vi "WS1050 36 DUT Reliability HD_Cycling Ver1.4.vi"() -> ()   [LabVIEW 2012]
uses:
  WS_VCAP Driver 029/Source/WSVCAP Shell/Type Defs/WSVCAP SHL I2C DUT Mask Mode Enum.ctl
  <vilib>/Utility/file.llb/Read From Spreadsheet File (DBL).vi
panel:
  out "VISA resource name out":refnum<visa-resource-name>="GPIB0::3::INSTR"
  out "error out 2":errorcluster={"status"=TRUE, "code"=-63192, "source"="niLvFpga_Open_PXI-7813R.vi"}
  in  "Reg1_Bit Cntrl":string[](array[string])=["01", "02", "04", "08", "10", "20", "40", "80", "03", "06", "0C", "D8", "33", "66", "CC", "07", "0E", "1C", "38", "70", "E0", "0F", "1E", "3C", "78", "F0", "1F", "3E", "7C", "F8", "3F", "7E", "FC", "7F", "FE", "FD", "FB", "F7", "EF", "DF", "BF", "7F", "FC", "F9", "F3", "E7", "CF", "9F", "3F", "F8", "F1", "E3", "C7", "8F", "1F", "F0", "E1", "C3", "87", "0F", "E0", "C1", "83", "07", "C0", "81", "03", "AA", "55", "00"]
  out "date string":string="5/19/2014"
  out "PS1 Out":refnum<visa-resource-name>
  out "Ke2000 Out":refnum<visa-resource-name>="GPIB0::9::INSTR"
  in  "VPI_Cmd":string[](array[string])=["00", "3B", "00"]
  in  "VPI Name":string[](array[string])=["All_Drivers OFF", "All Drivers ON", "All Drivers OFF2"]
  in  "Tab Control":T1(tab)
  in  "CP with DVA ON":i32(ring) items=["CP HDC 35V", "CP HDC 40.25V", "CP HDC 27.5V", "CP HDC 30.5V", "CP HDC 44V", "CP HDC 50V", "CP HDC 55V", "CP HDC 42.5V", "CP HDC 32V"]
  in  "No of Cmd":i64=2
  in  "Board#":string="BRD5"
  in  "Serial Number":string[][](table)=[["DUT", "SN"], ["DUT1", "1"], ["DUT2", "2"], ["DUT3", "3"], ["DUT4", "4"], ["DUT5", "5"], ["DUT6", "6"], ["DUT7", "7"], ["DUT8", "8"], ["DUT9", "9"], ["DUT10", "10"], ["DUT11", "11"], ["DUT12", "12"], ["DUT13", "13"], ["DUT14", "14"], ["DUT15", "15"], ["DUT16", "16"], ["DUT17", "17"], ["DUT18", "18"], ["DUT19", "19"], ["DUT20", "20"], ["DUT21", "21"], ["DUT22", "22"], ["DUT23", "23"], ["DUT24", "24"], ["DUT25", "25"], ["DUT26", "26"], ["DUT27", "27"], ["DUT28", "28"], ["DUT29", "29"], ["DUT30", "30"], ["DUT31", "31"], ["DUT32", "32"], ["DUT33", "33"], ["DUT34", "34"], ["DUT35", "35"], ["DUT36", "36"]]
  in  "SPI Clock Rate (Hz)":dbl=5000000.0 caption="Cycle Speed" format="%.1p Hz"
  in  "Wafer#":string="T7-EB"
  in  "File Name":string="CYC_WS1050_T7_EB_65C_40V_25DC_EMPTY_BRD5_151017_1"
  in  "TMN DC\\CAP Data Log File Path":path=path "C:/WS1050 36 DUT Data"
  in  "Test Program":string="WS1050 36 DUT Reliability HD_Cycling Ver1.4"
  out "Current Date":string="8/28/2014"
  out "Current Time":string="0950"
  in  "Start Date":string="10/21/2014"
  in  "Start Time":string="1542"
  in  "Comment":string="CYC65C40V"
  in  "OK Button":bool
  in  "Calibration":bool
  in  "Verify CP":bool
  in  "CP Setting":i32(ring) items=["CP OFF", "CP ON", "CP 35V", "CP 40V", "DVA ON", "DVA OFF", "REG1 ON", "REG1 OFF", "REG2 ON", "REG2 OFF", "REG3 ON", "REG3 OFF"]
  in  "Stop Calibration":bool
  in  "Set VDD":dbl=3.7 format="%.3g"
  in  "Command":string[](array[string])=["0702013B3B3B", "070201000000", "0702013B0000"]
  in  "Clock Rate (Hz)":dbl=1000000.0 caption="Meas Speed" format="%.1p Hz"
  out "AR  Measurent(Hz)":dbl
  in  "PS1 Source":refnum<visa-resource-name>="GPIB0::5::INSTR"
  in  "Ke2000":refnum<visa-resource-name>="GPIB0::9::INSTR"
  in  "CP to HD/Cycle":i32(ring)=1 items=["CP HDC 35V", "CP HDC 40.25V", "CP HDC 27.5V", "CP HDC 30.5V", "CP HDC 44V", "CP HDC 50V", "CP HDC 55V", "CP HDC 42.5V", "CP HDC 32V"]
  out "Simulate FPGA":bool
  out "Online":bool
  out "AR Cycling(Hz)":dbl=5000000.0
  in  "Ke2400":refnum<visa-resource-name>="GPIB0::3::INSTR"
  in  "Initialize AD7747":bool
  in  "DUT Mask Mode":T2=enum."All"
  in  "RFFE Slave Address":u8=7 caption="Slave Address" format="0x%02x"
  out "Activity Log":string="05/19/2014 -- 12:24:35.853::WSVCAP::APP::Application Started\n05/19/2014 -- 12:24:37.606::WSVCAP::WSVCAP SHL::WR I2C-REG:0x0A;MASK:0xFFFFFFFFFFFF;C1 DATA:22:22:22:22:22:22:22:22:22:22:22:22:22:22:22:22;C2 DATA:22:22:22:22:22:22:22:22:22:22:22:22:22:22:22:22;C3 DATA:22:22:22:22:22:22:22:22:22:22:22:22:22:22:22:22\r\n05/19/2014 -- 12:24:37.773::WSVCAP::WSVCAP SHL::WR I2C-ST:0,0,4,1\r\n05/19/2014 -- 12:24:37.903::WSVCAP::WSVCAP SHL::RD I2C-BYTES:4;ADD:0x00;MASK:0xFFFFFFFFFFFF\r\n05/19/2014 -- 12:24:38.045::WSVCAP::WSVCAP SHL::RD I2C:C1 DATA:2:2:2:2:2:2:2:2:2:2:2:2:2:2:2:2|A7:A9:AA:82:82:7F:82:81:82:81:83:82:81:82:82:81|46:36:BB:88:44:A3:E9:2B:32:20:ED:25:BB:3D:68:B|2C:6A:EB:A7:22:56:FE:CC:36:82:D7:B0:3B:48:F9:CC;C2 DATA:2:2:2:2:2:2:2:2:2:2:2:2:2:2:2:2|94:94:94:80:80:80:80:80:81:7E:7E:81:80:7E:80:80|47:33:15:82:62:B:E8:1C:D7:C3:7D:41:7C:B7:4C:2A|C4:B4:AE:8:1E:D1:4E:37:11:C0:6F:63:42:9D:63:B5;C3 DATA:2:2:2:2:2:2:2:2:2:2:2:2:2:2:2:2|95:95:95:81:81:7E:81:80:84:7D:80:83:81:7E:7F:80|AB:C4:14:B5:7B:52:DF:C9:79:5D:5F:30:99:31:1E:F4|6E:5C:F7:A8:C3:EB:7B:EF:33:92:89:77:4D:67:75:DD;STATUS:0:0:4:0\r\n05/19/2014 -- 12:24:38.046::WSVCAP::WSVCAP SHL::WR I2C-REG:0x0A;MASK:0xFFFFFFFFFFFF;C1 DATA:22:22:22:22:22:22:22:22:22:22:22:22:22:22:22:22;C2 DATA:22:22:22:22:22:22:22:22:22:22:22:22:22:22:22:22;C3 DATA:22:22:22:22:22:22:22:22:22:22:22:22:22:22:22:22\r\n05/19/2014 -- 12:24:38.089::WSVCAP::WSVCAP SHL::WR I2C-ST:0,0,4,1\r\n05/19/2014 -- 12:24:38.219::WSVCAP::WSVCAP SHL::RD I2C-BYTES:4;ADD:0x00;MASK:0xFFFFFFFFFFFF\r\n05/19/2014 -- 12:24:38.362::WSVCAP::WSVCAP SHL::RD I2C:C1 DATA:2:2:2:2:2:2:2:2:2:2:2:2:2:2:2:2|A7:AB:AA:82:82:82:83:83:82:82:82:82:7F:82:82:81|4B:32:96:83:3E:61:43:17:25:62:AB:4D:A2:40:2E:5|3C:76:2B:B4:EE:E4:A9:1A:AA:A:26:C7:21:2E:87:5B;C2 DATA:2:2:2:2:2:2:2:2:2:2:2:2:2:2:2:2|94:94:94:80:80:80:80:80:80:7F:80:81:80:80:7F:80|4A:32:19:7D:19:6C:79:46:61:7F:4B:B8:A5:30:F3:14|B4:70:A:8C:9C:DC:43:FA:1E:A:C6:21:A:A9:13:F3;C3 DATA:2:2:2:2:2:2:2:2:2:2:2:2:2:2:2:2|95:97:94:81:80:81:82:81:80:7E:81:84:7F:81:80:80|B2:32:D0:A7:9E:4C:AB:D4:EE:D9:F0:82:B7:91:7:FF|C1:91:B6:3D:D8:E:1B:4F:9F:6A:F1:6C:E7:3F:7:BA;STATUS:0:0:4:0\r\n05/19/2014 -- 12:24:38.364::WSVCAP::WSVCAP SHL::WR I2C-REG:0x0A;MASK:0xFFFFFFFFFFFF;C1 DATA:22:22:22:22:22:22:22:22:22:22:22:22:22:22:22:22;C2 DATA:22:22:22:22:22:22:22:22:22:22:22:22:22:22:22:22;C3 DATA:22:22:22:22:22:22:22:22:22:22:22:22:22:22:22:22\r\n05/19/2014 -- 12:24:38.406::WSVCAP::WSVCAP SHL::WR I2C-ST:0,0,4,1\r\n05/19/2014 -- 12:24:38.536::WSVCAP::WSVCAP SHL::RD I2C-BYTES:4;ADD:0x00;MASK:0xFFFFFFFFFFFF\r\n05/19/2014 -- 12:24:38.678::WSVCAP::WSVCAP SHL::RD I2C:C1 DATA:2:2:2:2:2:2:2:2:2:2:2:2:2:2:2:2|A7:A9:AB:82:82:81:82:82:82:82:82:82:82:82:82:81|46:71:4C:87:43:3D:7F:FC:25:4F:8E:54:97:3E:60:8C|AA:F4:1F:B5:CE:43:1F:36:9:87:9C:78:86:5:B6:8E;C2 DATA:2:2:2:2:2:2:2:2:2:2:2:2:2:2:2:2|94:94:94:80:7F:7F:80:80:80:80:80:81:80:80:80:80|49:36:18:7D:6E:C5:E4:3C:81:2E:41:D3:75:71:E3:72|E8:D3:E6:D1:E0:48:AE:D4:54:D:E8:8E:B4:41:68:4;C3 DATA:2:2:2:2:2:2:2:2:2:2:2:2:2:2:2:2|95:95:95:81:7F:7F:81:81:81:81:81:84:81:81:82:81|B3:F5:90:AB:82:69:7B:93:D0:77:E8:D5:E8:8C:84:E8|B9:AC:EE:2B:B6:71:8F:4A:74:31:56:BB:8A:B7:A0:C8;STATUS:0:0:4:0\r\n05/19/2014 -- 12:24:38.681::WSVCAP::WSVCAP SHL::WR I2C-REG:0x0A;MASK:0xFFFFFFFFFFFF;C1 DATA:22:22:22:22:22:22:22:22:22:22:22:22:22:22:22:22;C2 DATA:22:22:22:22:22:22:22:22:22:22:22:22:22:22:22:22;C3 DATA:22:22:22:22:22:22:22:22:22:22:22:22:22:22:22:22\r\n05/19/2014 -- 12:24:38.723::WSVCAP::WSVCAP SHL::WR I2C-ST:0,0,4,1\r\n05/19/2014 -- 12:24:38.854::WSVCAP::WSVCAP SHL::RD I2C-BYTES:4;ADD:0x00;MASK:0xFFFFFFFFFFFF\r\n05/19/2014 -- 12:24:38.996::WSVCAP::WSVCAP SHL::RD I2C:C1 DATA:2:2:2:2:2:2:2:2:2:2:2:2:2:2:2:2|A7:A9:AA:82:82:7F:83:81:82:81:84:82:7F:82:7F:82|43:FB:E:7F:3C:AD:35:35:26:A2:6C:21:4B:3D:8:6|63:9A:E1:F3:95:32:91:42:90:3C:78:1F:5C:D7:5F:D8;C2 DATA:2:2:2:2:2:2:2:2:2:2:2:2:2:2:2:2|94:94:94:80:80:80:80:80:81:80:7E:81:80:7E:7F:80|48:36:18:7F:5E:3D:69:83:DE:AE:A1:9E:31:AE:BB:96|15:A0:44:17:13:FD:CC:C8:6D:B2:EF:A7:C:C7:3B:F;C3 DATA:2:2:2:2:2:2:2:2:2:2:2:2:2:2:2:2|95:96:94:81:81:7E:82:80:84:80:80:84:7F:7E:7D:82|AD:3B:6D:A9:7C:57:9D:F5:7A:96:23:5C:36:2D:ED:5A|CD:46:DB:3B:C7:BD:70:60:33:B8:B:F7:63:A:51:4D;STATUS:0:0:4:0\r\n05/19/2014 -- 12:24:38.998::WSVCAP::WSVCAP SHL::WR I2C-REG:0x0A;MASK:0xFFFFFFFFFFFF;C1 DATA:22:22:22:22:22:22:22:22:22:22:22:22:22:22:22:22;C2 DATA:22:22:22:22:22:22:22:22:22:22:22:22:22:22:22:22;C3 DATA:22:22:22:22:22:22:22:22:22:22:22:22:22:22:22:22\r\n05/19/2014 -- 12:24:39.040::WSVCAP::WSVCAP SHL::WR I2C-ST:0,0,4,1\r\n05/19/2014 -- 12:24:39.170::WSVCAP::WSVCAP SHL::RD I2C-BYTES:4;ADD:0x00;MASK:0xFFFFFFFFFFFF\r\n05/19/2014 -- 12:24:39.311::WSVCAP::WSVCAP SHL::RD I2C:C1 DATA:2:2:2:2:2:2:2:2:2:2:2:2:2:2:2:2|A7:AA:AB:82:82:81:82:81:82:81:82:82:82:82:7F:82|44:F1:90:87:45:44:C8:2C:2C:F1:FC:1B:94:3B:3C:75|4A:49:95:19:99:73:64:3:23:24:F3:A2:5E:7F:C4:B6;C2 DATA:2:2:2:2:2:2:2:2:2:2:2:2:2:2:2:2|94:94:94:80:80:80:80:7F:80:80:7E:80:80:7E:7F:80|4C:36:17:7D:A8:9F:DE:C7:53:6D:8A:F4:41:A5:C6:E0|90:2E:24:C:D9:22:E4:76:3B:40:1D:53:33:B1:3E:4D;C3 DATA:2:2:2:2:2:2:2:2:2:2:2:2:2:2:2:2|95:97:95:81:81:7F:81:80:80:81:7F:82:81:7E:7D:82|AE:2B:A7:AB:CC:CD:A4:38:FD:17:80:F2:92:2D:45:C4|76:E5:D:B9:AD:B5:BA:8D:28:32:9E:42:B7:20:4A:D9;STATUS:0:0:4:0\r\n05/19/2014 -- 12:24:39.313::WSVCAP::WSVCAP SHL::WR I2C-REG:0x0A;MASK:0xFFFFFFFFFFFF;C1 DATA:22:22:22:22:22:22:22:22:22:22:22:22:22:22:22:22;C2 DATA:22:22:22:22:22:22:22:22:22:22:22:22:22:22:22:22;C3 DATA:22:22:22:22:22:22:22:22:22:22:22:22:22:22:22:22\r\n05/19/2014 -- 12:24:39.355::WSVCAP::WSVCAP SHL::WR I2C-ST:0,0,4,1\r\n05/19/2014 -- 12:24:39.486::WSVCAP::WSVCAP SHL::RD I2C-BYTES:4;ADD:0x00;MASK:0xFFFFFFFFFFFF\r\n05/19/2014 -- 12:24:39.628::WSVCAP::WSVCAP SHL::RD I2C:C1 DATA:2:2:2:2:2:2:2:2:2:2:2:2:2:2:2:2|A7:A9:AA:82:82:82:83:82:82:82:82:82:7F:82:7F:82|47:18:E4:87:3E:E7:6:65:25:92:37:38:A8:3E:89:85|7C:A7:7:2B:A3:7A:EC:EF:89:ED:F4:D3:D8:BC:3A:F5;C2 DATA:2:2:2:2:2:2:2:2:2:2:2:2:2:2:2:2|94:94:94:80:7F:80:80:7F:81:80:7E:80:80:80:81:80|49:37:17:80:76:25:6A:F8:DF:55:97:4D:B8:5B:2B:B1|13:E3:9A:3E:1A:2D:4F:B6:DB:E9:61:FA:8B:D6:9:CC;C3 DATA:2:2:2:2:2:2:2:2:2:2:2:2:2:2:2:2|95:95:95:81:7F:80:82:81:84:80:7F:81:80:81:7F:82|AF:93:3B:AF:5B:11:82:E4:7E:C3:2D:72:9:96:D9:A|DB:96:F2:10:5F:64:9A:C6:98:12:27:7D:10:D3:20:D9;STATUS:0:0:4:0\r\n05/19/2014 -- 12:24:40.132::WSVCAP::WSVCAP SHL::CLOSE\r\n"
  in  "C1 Cap DAC":u8=128 caption="B Data In" format="0x%02x"
  in  "C2 Cap DAC":u8=128 caption="B Data In" format="0x%02x"
  in  "C3 Cap DAC":u8=128 caption="B Data In" format="0x%02x"
  out "IDD Brd(uA)":string
  in  "Repeat Meas(s)":u32=900
  in  "Real No. From\nLookup Table":bool
  in  "Control Panel":T3={"Verify Socket"=FALSE, "HD/CYC"=FALSE, "E-CAL"=FALSE, "DVA"=FALSE, "VPI"=TRUE, "VSA"=TRUE, "HS"=TRUE}
  out "Verify Socket":bool
  out "HD/CYC":bool
  out "E-CAL":bool
  out "DVA":bool
  out "VPI":bool
  out "VSA":bool
  out "HS":bool
  in  "Lot#":string="WS1050"
  out "AD7747 Values":string[][](table)
  in  "Freq(Hz)":string="12K"
  in  "Reset P/S":bool
  in  "Test Sequences":i32(ring) items=["C1_C2_C3", "C2_C1_C3", "C3_C2_C1"]
  in  "WS1050/51":bool=TRUE
  in  "% Duty Cycle":string="25"
  in  "Cmd To HD":string="0702013B3B3B"
  in  "Post CMd Delay":dbl[](array[numeric])=[1.7e-05, 5.4e-05, 1.8e-05] min=0.0 max=0.5 format="%#.0p s"
  in  "Cmin/Act":bool=TRUE
  in  "CP to Meas":i32(ring)=1 items=["CP HDC 35V", "CP HDC 40.25V", "CP HDC 27.5V", "CP HDC 30.5V", "CP HDC 44V", "CP HDC 50V", "CP HDC 55V", "CP HDC 42.5V", "CP HDC 32V"]
  in  "CP VPI":i32(ring) items=["CP HDC 35V", "CP HDC 40.25V", "CP HDC 27.5V", "CP HDC 30.5V", "CP HDC 44V", "CP HDC 50V", "CP HDC 55V", "CP HDC 42.5V", "CP HDC 32V"]
  out "CAP_C1":string[][](table)
  out "NOM IDD OFF(uA)":string
  out "CAP_C2":string[][](table)
  out "CAP_C3":string[][](table)
  out "Total Time":u64
  in  "Set HD/Cycle \nto Complete":u64=5000000000
  out "No of HD/Cycle\nCompleted":u64
  out "Cycle Count":u64 min=1 max=4 step=1
  out "Loop \ncompleted":i32=1
  out "Previous Time":string="12:20:26 PM"
  out "STATUS":string="Idle...."
  out "Total Delta C2(pF)":string[](array[string])
  out "Total Delta C1(pF)":string[](array[string])
  out "Total Delta C3(pF)":string[](array[string])
  out "RB Reg for HD":string[](array[string])
  out "RB Reg for HD/Cycle":string[](array[string])
  out "VPI C2":string[][](table)
  out "VPI C3":string[][](table)
  out "NOM IDD ON (uA)":string
  out "IDD_HD/CYC (uA)":string="164.601255E+0"
  in  "stop During HD/Cycles":bool
  in  "stop":bool
  out "IDD Stdby(uA)":string="2.606990E+0"
  out "VPI C1":string[][](table)
  out "VSA_V1":string[][](table)
  out "VSA_V2":string[][](table)
  out "VSA_V3":string[][](table)
  in  "VSA Voltage(V)":dbl[](array[numeric])=[-10.0, 0.0, 10.0]
  in  "DC_Temp":i32=65
  in  "HD/CYC Temp":i32=65
  in  "Time All ON (s)":u32=120
  in  "Time All OFF (s)":u32=120
  in  "HD_DC (Min)":u64=259200
  out "LPs Count":i32
  in  "X Repeat":i32=100
  out "No LPs to RP":i32
  out "Run Loops":i32=1
  out "TTCompleted":u64=2000
  in  "TTF Completed":u64=5000000000
  out "% Delta C_T0":string[][](array[string])
  out "% Delta C":string[][](array[string])
  out "EFuse RB T0":string[](array[string])
  out "Current EFuse Read back":string[](array[string])
  out "EFuse Readback Status":bool[](array[boolean])
  in  "DeltaC Target Setting(pF)":dbl=7.375
  out "error out":errorcluster
  in  "error in (no error)":errorcluster
  in  "HD RP":dbl=60.0
  in  "Cycle RP":dbl=10000.0
  out "Min Plot_1":dbl[][](graph) caption="(Y) Multi Plot 2"
  out "Min Plot_2":dbl[][](graph) caption="(Y) Multi Plot 2"
  out "Min Plot_3":dbl[][](graph) caption="(Y) Multi Plot 2"
  in  "Debug":bool
  in  "No of Rows\nFrom Spread Sheet":i32
  in  "Plot Delta Cmin":bool=TRUE
  in  "Plot":T4(ring)
  in  "Bank C1":i32(ring) items=["C1", "C2", "C3", "D_C1", "D_C2", "D_C3"]
  in  "Bank C2":i32(ring)=1 items=["C1", "C2", "C3", "D_C1", "D_C2", "D_C3"]
  in  "Bank C3":i32(ring)=2 items=["C1", "C2", "C3", "D_C1", "D_C2", "D_C3"]
  # "Company:  WiSpry Inc\n20 Fairbanks Ste 198 Irvine CA 92618\n\nAuthor:  Andy V Tran\nCreated:  08/07/2015\nLabVIEW 2012 Pro\nTest Program:  WS1050 36 DUT Reliability HD_Cycling ver1.4\nFPGA: WS_VCAP Driver 029"
  # "Note for HD Duty Cycle:\n1.  Set time to start HD_DC (Min), default is 259200 (6 months) \n2.  Set Time for Duty Cycle ON/OFF, default setting is 2 minutes\n3.  No of Loops to RP = 3600s/(Time ALL ON(s) + Time ALL + OFF(s))\n4.  Set X Repeat = no of runs, default is 100 runs\n5.  Set TTF Completed to stop the test.\n\nVer 1.4 updated based on Ver1.3:\n1.  Updated P/S E3631A Driver\n2.  Updated KE2400 Driver\n3.  Updated CP to HD/Cycle"
  # "Minutes"
  # "X1000"
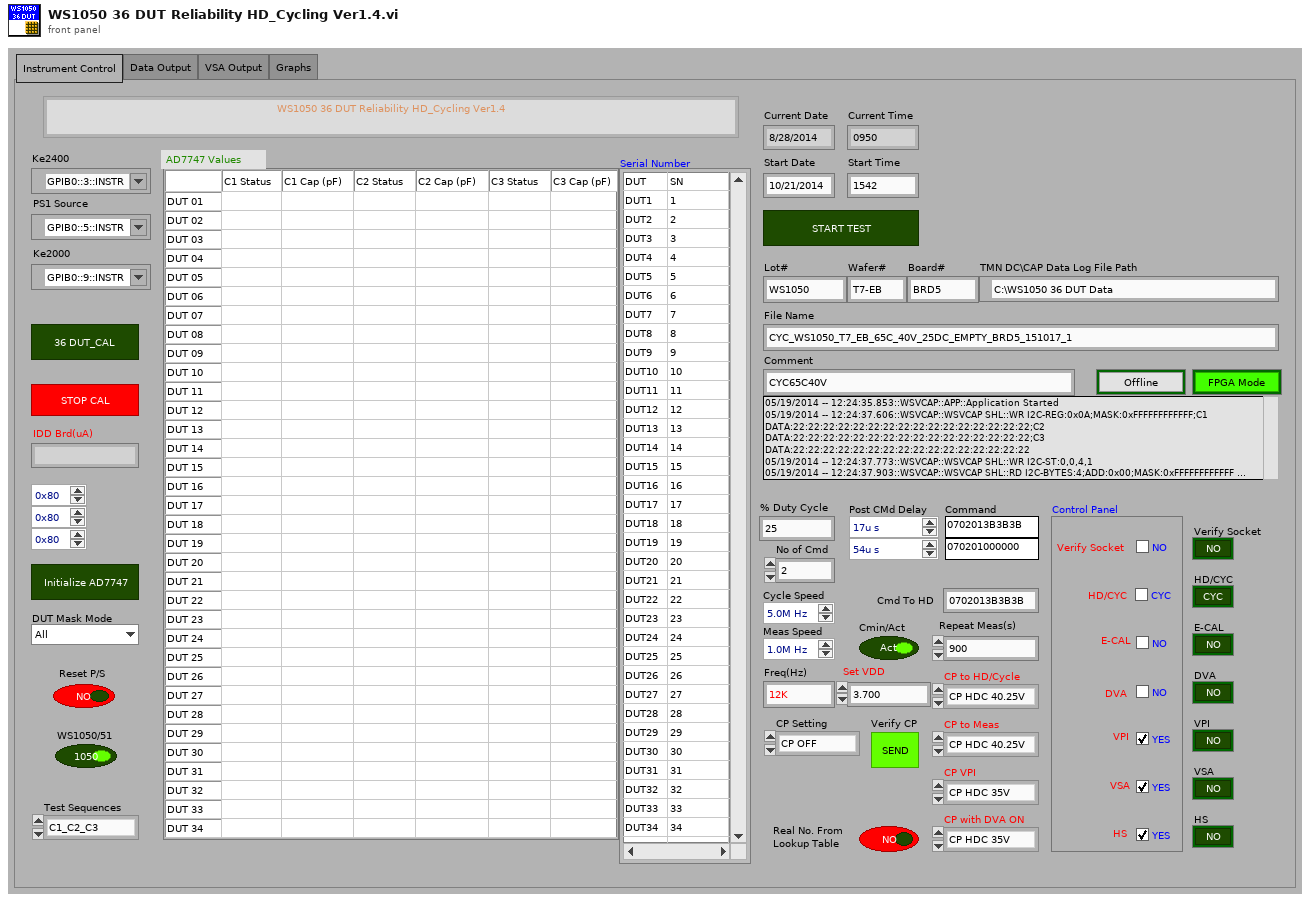
[diagram p1: front panel]
types:
  T1 = enum32{"Instrument Control", "Data Output", "VSA Output", "Graphs"}
  T2 = typedef "WSVCAP SHL I2C DUT Mask Mode Enum.ctl" = enum16{"Custom", "C1", "C2", "C3", "All"}
  T3 = cluster{"Verify Socket":bool, "HD/CYC":bool, "E-CAL":bool, "DVA":bool, "VPI":bool, "VSA":bool, "HS":bool}
  T4 = enum16{"ALL DUTs", "DUT 01", "DUT 02", "DUT 03", "DUT 04", "DUT 05", "DUT 06", "DUT 07", "DUT 08", "DUT 09", "DUT 10", "DUT 11", "DUT 12", "DUT 13", "DUT 14", "DUT 15", "DUT 16", "DUT 17", "DUT 18", "DUT 19", "DUT 20", "DUT 21", "DUT 22", "DUT 23", "DUT 24", "DUT 25", "DUT 26", "DUT 27", "DUT 28", "DUT 29", "DUT 30", "DUT 31", "DUT 32", "DUT 33", "DUT 34", "DUT 35", "DUT 36"}
  T5 = typedef "WSVCAP SHL Core System Cluster.ctl" = cluster{"Settings":T6, "FPGA Resource":tag, "Online":bool, "I2C Wait Ticks":u32, "SPI Wait Ticks":u32, "RFFE Wait Ticks":u32}
  T6 = typedef "WSVCAP SHL I2C Settings Cluster.ctl" = cluster{"FPGA Resource Name":string, "I2C Slave Address":u8, "I2C Clock Rate (Hz)":dbl, "SPI Clock Rate (Hz)":dbl, "RFFE Slave Address":u8, "RFFE Clock Rate (Hz)":dbl, "Simulate FPGA":bool, "C1 Cap DAC Default":u8, "C2 Cap DAC Default":u8, "C3 Cap DAC Default":u8}
  T7 = enum16{"Idle...", "Voltage 1", "Voltage 2", "Voltage 3"}[]
  T8 = cluster{"Test Program ":string, "Comment":string, "Data Out":string, "Data Out":string, "Data Out":string, string, "Data Out":string, "Data Out":string, "Data Out":string, "Freq(Hz)":string, "Board#":string}
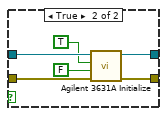
[diagram p2: hidden frame]
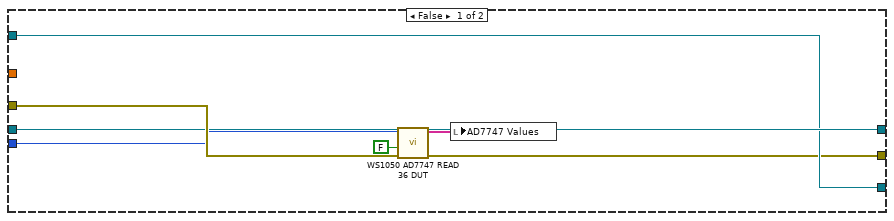
[diagram p10: hidden frame]
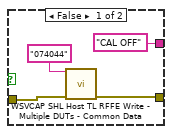
[diagram p11: hidden frame]
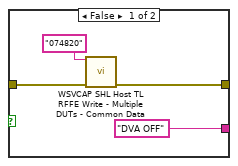
[diagram p12: hidden frame]
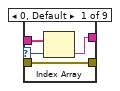
[diagram p13: hidden frame]
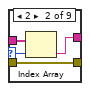
[diagram p14: hidden frame]
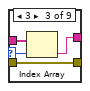
[diagram p15: hidden frame]
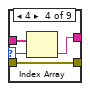
[diagram p16: hidden frame]
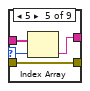
[diagram p17: hidden frame]
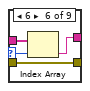
[diagram p18: hidden frame]
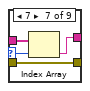
[diagram p19: hidden frame]
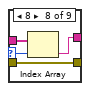
[diagram p20: hidden frame]
diagram:
  w25 = TRUE
  w29 = u16 0 items=["Off", "Moving Filter", "Repeating Filter"] ("Digital Filter (0: Off)")
  w30 = u16 7 items=["3.5 Digits"=4, "4.5 Digits"=5, "5.5 Digits"=6, "6.5 Digits"=7] ("Resolution (7: 6.5 digits)")
  n1 = case shown="True" w25 {
    tunnel: "error in (no error)" -> [w37 w38]
    tunnel: [w37 w45] -> w14
    frame False {
    }
    frame True {
      n2 = call "WSVCAP SHL Host TL Initialize.vi"("error in"=w38) -> ("error out"=w39:errorcluster)  [unwired: 13 in, 1 out]
      n3 = control-ref of="Activity Log"() -> (w41:refnum<vi>)
      n4 = call "ACT LG Activity Log Core.vi"("Display Ref"=w41, "Source"="WSVCAP", "Error In (no error)"=w39) -> ("Error Out"=w40:errorcluster)  [unwired: 11 in, 1 out]
      n5 = call "WSVCAP SHL Host TL Status Manager.vi"("error in"=w40) -> ("System Out"=w46:T5, "error out"=w45:errorcluster)  [unwired: 13 in]
      n6 = Unbundle By Name(w46) -> ("Online"=→"Online":bool, "Settings.Simulate FPGA"=→"Simulate FPGA":bool)
    }
  }
  n7 = case shown="True" TRUE {
    tunnel: w14 -> [w47 w52]
    tunnel: [w48 w51] -> w22
    tunnel: [w47 w50] -> w18
    tunnel: "Ke2400" -> [w48 w49]
    frame False {
    }
    frame True {
      n8 = VISA Write(VISA resource name=w49, write buffer="SOUR:FUNC VOLT;VOLT:MODE FIX;RANG 100;LEV 0.0;:SENS:FUNC \"CURR\";CURR:PROT 60E-3;RANG 100E-3;:OUTP ON", error in (no error)=w52) -> (VISA resource name out=w51:refnum<visa-resource-name>, error out=w50:errorcluster)  [unwired: 1 out]
    }
  }
  n9 = case shown="False" "Reset P/S" {
    tunnel: "PS1 Source" -> [w54 w61]
    tunnel: [w54 w59] -> w34
    tunnel: w14 -> [w55 w57]
    tunnel: [w55 w56] -> w13
    frame False {
    }
    frame True {
      n10 = call "Agilent 3631A Initialize.vi"("error in (no error)"=w57, "Default"=FALSE ("Reset? (T: Yes)"), "Reset"=TRUE ("ID Query? (T: Yes)"), "VISA resource name"=w61) -> ("error out"=w56:errorcluster, "VISA resource name out"=w59:refnum<visa-resource-name>)  [unwired: 6 in]
    }
  }
  n11 = call "Ke2000 Initialize.vi"("error in (no error)"=w14, "VISA resource name"="Ke2000") -> ("error out"=w31:errorcluster, "VISA resource name out"=w32:refnum<visa-resource-name>)  [unwired: 8 in]
  n12 = call "Ke2000 Configure DC Current.vi"("Resolution (7: 6.5 digits)"=w30, "Digital Filter (0: Off)"=w29, "Auto Range? (T: Auto)"=FALSE, "error in"=w31, "Custom Range (0 A)"=1.0, "VISA resource name"=w32) -> ("error out"=w15:errorcluster, "VISA resource name out"=w27:refnum<visa-resource-name>)  [unwired: 4 in]
  n13 = case shown="True" TRUE {
    tunnel: [_ w62] -> w36
    frame False {
    }
    frame True {
      n14 = call-poly <vilib>:"Read From Spreadsheet File.vi"("number of rows (all:-1)"=-1) -> ("all rows"=w62:dbl[][])  [unwired: 6 in, 4 out]
    }
  }
  n15 = Merge Errors(w18, w15, w13) -> (w23:errorcluster)
  n16 = while {
    tunnel: w23 -> [w70]
    tunnel: [w66] -> w4
    tunnel: w36 -> [w93]
    tunnel: w34 -> [w81]
    tunnel: w27 -> [w82]
    tunnel: [w91] -> w10
    tunnel: [w90] -> w5
    tunnel: w22 -> [w88]
    tunnel: [w87] -> w20
    tunnel: [FALSE ("stop")] -> w16
    i -> [w89]
    stop <- w94 stop-if-true
    n17 = case shown="0" w89 {
      tunnel: w70 -> [w104 w106]
      tunnel: [w103 w106] -> w84
      tunnel: "RFFE Slave Address" -> [w101 _]
      frame 0 {
        w97 = dbl[][] []
        w96 = "" ("uA")
        w98 = string[][] []
        w99 = string[] [] ("EFuse Read back")
        w105 = u64 0 ("No of HD/Cycle\nCompleted")
        n18 = local write "RB Reg for HD/Cycle"(w99) -> ()
        n19 = local write "Current EFuse Read back"(w99) -> ()
        n20 = local write "EFuse RB T0"(w99) -> ()
        n21 = local write "Total Delta C1(pF)"(w99) -> ()
        n22 = local write "Total Delta C2(pF)"(w99) -> ()
        n23 = local write "Total Delta C3(pF)"(w99) -> ()
        n24 = local write "No of HD/Cycle\nCompleted"(w105) -> ()
        n25 = local write "Cycle Count"(w105) -> ()
        n26 = local write "CAP_C2"(w98) -> ()
        n27 = local write "CAP_C1"(w98) -> ()
        n28 = local write "VPI C2"(w98) -> ()
        n29 = local write "VSA_V3"(w98) -> ()
        n30 = local write "VSA_V1"(w98) -> ()
        n31 = local write "NOM IDD OFF(uA)"(w96) -> ()
        n32 = local write "NOM IDD ON (uA)"(w96) -> ()
        n33 = local write "IDD Brd(uA)"(w96) -> ()
        n34 = local write "CAP_C3"(w98) -> ()
        n35 = local write "VSA_V2"(w98) -> ()
        n36 = local write "VPI C1"(w98) -> ()
        n37 = local write "VPI C3"(w98) -> ()
        n38 = local write "% Delta C"(w98) -> ()
        n39 = local write "% Delta C_T0"(w98) -> ()
        n40 = call "WSVCAP SHL Host TL RFFE Configure.vi"("RFFE Slave Address"=w101, "Clock Rate (Hz)"="Clock Rate (Hz)", "error in"=w104) -> ("Actual Rate (Hz)"=→"AR  Measurent(Hz)":dbl, "error out"=w103:errorcluster)  [unwired: 11 in]
        n41 = local write "Min Plot_3"(w97) -> ()
        n42 = local write "Min Plot_1"(w97) -> ()
        n43 = local write "Min Plot_2"(w97) -> ()
      }
      frame 1, Default {
      }
    }
    n44 = while {
      tunnel: ["stop"] -> w86
      tunnel: w84 -> [w134]
      tunnel: [w126] -> w78
      tunnel: w81 -> [w133]
      tunnel: w82 -> [w128]
      tunnel: [w129] -> w80
      tunnel: [w127] -> w79
      tunnel: [w124] -> w77
      tunnel: [w123] -> w76
      tunnel: [w122] -> w75
      tunnel: [w121] -> w74
      tunnel: [w120] -> w73
      tunnel: [w119] -> w72
      tunnel: [w118] -> w71
      tunnel: ["Command"] -> w69
      tunnel: ["Post CMd Delay"] -> w68
      tunnel: "Set VDD" -> [w108]
      stop <- w141 stop-if-true
      # "Set Date & Time to Start Test"
      n45 = case shown="True" "Initialize AD7747" {
        tunnel: w134 -> [w150 w156]
        tunnel: [w150 w152] -> w117
        tunnel: w133 -> [w149 w154]
        tunnel: [w149 w153] -> w132
        tunnel: w108 -> [_ w151]
        frame False {
        }
        frame True {
          w157 = T7 [enum."Voltage 2", enum."Voltage 3", enum."Voltage 1"] items=["Idle...", "Voltage 1", "Voltage 2", "Voltage 3"]
          n46 = for {
            tunnel: w154 -> [w167]
            tunnel: w157 -> [w165] mode=indexing
            tunnel: [w164] -> w153
            shift-right: [w161] -> w155
            shift-left: w156 -> [w168]
            tunnel: w151 -> [w158]
            n47 = call "E3631A_Voltage Controller updated.vi"("VISA resource name"=w167, "I_VDD(A)"=0.5, "Channel Controller"=w165, "Voltage 1"=w158, "Voltage 2"=3.3, "error in (no error)"=w168, "I_3.3V (A)"=0.5) -> ("VISA resource name out"=w164:refnum<visa-resource-name>, "error out"=w160:errorcluster)  [unwired: 7 in]
            n48 = call "Delay.vi"("milliseconds to wait"=u32 100, "error in (no error)"=w160) -> ("error out"=w161:errorcluster)  [unwired: 9 in]
          }
          n49 = call "WS1050_AD7747_Init 36DUT.vi"("error in"=w155) -> ("error out"=w152:errorcluster)  [unwired: 10 in]
        }
      }
      n50 = call "Time_stamp.vi"() -> ("date/time string"=w146:string, "date string"=w148:string)  [unwired: 2 in]
      "Current Date" <- w148
      "Current Time" <- w146
      n51 = Equal?(x=w148, y="Start Date") -> (x = y?=w144:bool)
      n52 = Equal?(x=w146, y="Start Time") -> (x = y?=w143:bool)
      n53 = And(x=w144, y=w143) -> (x .and. y?=w140:bool)
      n54 = Compound Arithmetic op=OR(w140, "OK Button", "stop") -> (w141:bool)
      n55 = case shown="True" "Calibration" {
        tunnel: w117 -> [w199 w217]
        tunnel: [w193 w214] -> w115
        tunnel: w132 -> [w198 w213]
        tunnel: "DUT Mask Mode" -> [w197 w209]
        tunnel: [w198 w208] -> w130
        tunnel: w128 -> [w196 w204]
        tunnel: [w196 w201] -> w127
        tunnel: w108 -> [_ w200]
        frame False {
          n56 = call "WS1050 AD7747 READ 36 DUT.vi"("error in"=w199, "Log (T)"=FALSE, "DUT Mask Mode (All)"=w197) -> ("error out"=w193:errorcluster, "AD7747 Values"=w194:string[][])  [unwired: 7 in]
          n57 = local write "AD7747 Values"(w194) -> ()
        }
        frame True {
          n58 = flat-sequence {
            tunnel: w217 -> [w227]
            tunnel: [w222] -> w216
            tunnel: w213 -> [w226]
            tunnel: [w225] -> w212
            tunnel: w209 -> [w224]
            tunnel: [w224] -> w210
            tunnel: w204 -> [w220]
            tunnel: [w219] -> w203
            tunnel: w200 -> [w218]
            tunnel: w216 -> [w251]
            tunnel: [w250] -> w215
            tunnel: w212 -> [w249]
            tunnel: [w249] -> w211
            tunnel: w210 -> [w248]
            tunnel: "C1 Cap DAC" -> [w244]
            tunnel: "C2 Cap DAC" -> [w243]
            tunnel: "C3 Cap DAC" -> [w242]
            tunnel: w203 -> [w241]
            tunnel: [w241] -> w202
            tunnel: w215 -> [w260]
            tunnel: [w263] -> w214
            tunnel: w211 -> [w262]
            tunnel: [w259] -> w208
            tunnel: w202 -> [w258]
            tunnel: [w258] -> w201
            frame #0 {
              w228 = T7 [enum."Voltage 2", enum."Voltage 3", enum."Voltage 1"] items=["Idle...", "Voltage 1", "Voltage 2", "Voltage 3"]
              n59 = for {
                tunnel: w226 -> [w239]
                tunnel: w228 -> [w237] mode=indexing
                tunnel: [w236] -> w225
                shift-right: [w234] -> w221
                shift-left: w227 -> [w240]
                tunnel: w218 -> [w230]
                n60 = call "E3631A_Voltage Controller updated.vi"("VISA resource name"=w239, "I_VDD(A)"=0.5, "Channel Controller"=w237, "Voltage 1"=w230, "Voltage 2"=3.3, "error in (no error)"=w240, "I_3.3V (A)"=0.5) -> ("VISA resource name out"=w236:refnum<visa-resource-name>, "error out"=w233:errorcluster)  [unwired: 7 in]
                n61 = call "Delay.vi"("milliseconds to wait"=u32 100, "error in (no error)"=w233) -> ("error out"=w234:errorcluster)  [unwired: 9 in]
              }
              n62 = call "Ke2000 Single Reading.vi"("error in (no error)"=w221, "VISA resource name"=w220) -> ("error out"=w222:errorcluster, "VISA resource name out"=w219:refnum<visa-resource-name>, "uA"=→"IDD Brd(uA)":string)  [unwired: 5 in, 2 out]
              n63 = One Button Dialog(message="Please verify all sockets should be empty...") -> ()  [unwired: 1 in, 1 out]
            }
            frame #1 {
              n64 = call "WS1050 CAPDAC Setting.vi"("DUT Mask Mode (All)"=w248, "error in"=w251, "C3 Cap DAC"=w242, "C2 Cap DAC"=w243, "C1 Cap DAC"=w244) -> ("error out"=w246:errorcluster)  [unwired: 5 in, 1 out]
              n65 = call "WS1050 OFFSET CAL.vi"("error in"=w246, "OFFSET CAL"=TRUE ("Read?")) -> ("error out"=w245:errorcluster)  [unwired: 8 in, 1 out]
              n66 = while {
                tunnel: w245 -> [w257]
                tunnel: [w256] -> w250
                tunnel: w248 -> [w254]
                stop <- "Stop Calibration" stop-if-true
                n67 = call "WS1050 AD7747 READ 36 DUT.vi"("error in"=w257, "Log (T)"=FALSE, "DUT Mask Mode (All)"=w254) -> ("error out"=w256:errorcluster, "AD7747 Values"=→"AD7747 Values":string[][])  [unwired: 7 in]
              }
            }
            frame #2 {
              w261 = T7 [enum."Voltage 2", enum."Voltage 3", enum."Voltage 1"] items=["Idle...", "Voltage 1", "Voltage 2", "Voltage 3"]
              n68 = for {
                tunnel: w262 -> [w275]
                tunnel: w261 -> [w272] mode=indexing
                tunnel: [w271] -> w259
                shift-right: [w267] -> w263
                shift-left: w260 -> [w273]
                n69 = call "E3631A_Voltage Controller updated.vi"("VISA resource name"=w275, "I_VDD(A)"=0.5, "Channel Controller"=w272, "Voltage 1"=0.0, "Voltage 2"=3.3, "error in (no error)"=w273, "I_3.3V (A)"=0.5) -> ("VISA resource name out"=w271:refnum<visa-resource-name>, "error out"=w266:errorcluster)  [unwired: 7 in]
                n70 = call "Delay.vi"("milliseconds to wait"=u32 100, "error in (no error)"=w266) -> ("error out"=w267:errorcluster)  [unwired: 9 in]
              }
              n71 = One Button Dialog(message="Calibration Completed....") -> ()  [unwired: 1 in, 1 out]
            }
          }
        }
      }
      n72 = local write "stop During HD/Cycles"(FALSE ("stop During HD/Cycles")) -> ()
      n73 = call "Control Panel.vi"("error in (no error)"=w117, "Control Panel"="Control Panel") -> ("error out"=w114:errorcluster, "VPI"=w120:bool, "DVA"=w121:bool, "E-CAL"=w122:bool, "VSA"=w119:bool, "HD/CYC"=w123:bool, "HS"=w118:bool, "Verify Socket"=w124:bool)  [unwired: 2 in]
      "Verify Socket" <- w124
      "E-CAL" <- w122
      "VPI" <- w120
      "VSA" <- w119
      "HS" <- w118
      "HD/CYC" <- w123
      "DVA" <- w121
      n74 = Merge Errors(w114, w115) -> (w116:errorcluster)
      n75 = case shown="True" "Verify CP" {
        tunnel: [w169 w174] -> w126
        tunnel: w130 -> [w170 w177]
        tunnel: [w170 w175] -> w129
        tunnel: w116 -> [w169 w173]
        tunnel: w108 -> [_ w171]
        frame False {
        }
        frame True {
          w178 = T7 [enum."Voltage 2", enum."Voltage 3", enum."Voltage 1"] items=["Idle...", "Voltage 1", "Voltage 2", "Voltage 3"]
          # "Verify CP"
          n76 = for {
            tunnel: w177 -> [w191]
            tunnel: w178 -> [w189] mode=indexing
            shift-right: [w187] -> w176
            shift-left: w173 -> [w192]
            tunnel: [w185] -> w175
            tunnel: w171 -> [w182]
            n77 = call "E3631A_Voltage Controller updated.vi"("VISA resource name"=w191, "I_VDD(A)"=0.5, "Channel Controller"=w189, "Voltage 1"=w182, "Voltage 2"=3.3, "error in (no error)"=w192, "I_3.3V (A)"=0.5) -> ("VISA resource name out"=w185:refnum<visa-resource-name>, "error out"=w188:errorcluster)  [unwired: 7 in]
            n78 = call "Delay.vi"("milliseconds to wait"=u32 100, "error in (no error)"=w188) -> ("error out"=w187:errorcluster)  [unwired: 9 in]
          }
          n79 = Index Array(array=string[] ["074000", "074040", "07476F", "074776", "074800", "074820", "07413B", "074100", "07423B", "074200", "07433B", "074300"], index="CP Setting") -> (element=w179:string)
          n80 = call "WSVCAP SHL Host TL RFFE Write - Multiple DUTs - Common Data.vi"("Data Out"=w179, "error in"=w176, "Log (T)"=FALSE) -> ("error out"=w174:errorcluster)  [unwired: 12 in]
        }
      }
      n81 = Array Subset(array="Post CMd Delay", length="No of Cmd") -> (w112:dbl[])  [unwired: 1 in]
      n82 = Array Subset(array="Command", length="No of Cmd") -> (w113:string[])  [unwired: 1 in]
      n83 = property on="Post CMd Delay" class="Arr (strict)"("Number of Rows"="No of Cmd") -> ()  [unwired: 2 in, 2 out]
      n84 = local write "Command"(w113) -> ()
      n85 = local write "Post CMd Delay"(w112) -> ()
      n86 = property on="Command" class="Arr (strict)"("Number of Rows"="No of Cmd") -> ()  [unwired: 2 in, 2 out]
      n87 = Wait Until Next ms Multiple(millisecond multiple=u32 100) -> ()  [unwired: 1 out]
    }
    n88 = case shown="False" w86 {
      tunnel: w78 -> [w336 w2007]
      tunnel: [w321 w2007] -> w66
      tunnel: w93 -> [w337 _]
      tunnel: w80 -> [w335 w2005]
      tunnel: w79 -> [w327 w2006]
      tunnel: [w333 w2006] -> w91
      tunnel: [w331 w2005] -> w90
      tunnel: w88 -> [w324 w2004]
      tunnel: [w320 w2004] -> w87
      tunnel: "RFFE Slave Address" -> [w315 _]
      tunnel: [FALSE ("stop During HD/Cycles") FALSE ("stop During HD/Cycles")] -> _
      tunnel: w77 -> [w291 _]
      tunnel: w76 -> [w290 _]
      tunnel: w75 -> [w289 _]
      tunnel: w74 -> [w288 _]
      tunnel: w73 -> [w287 _]
      tunnel: w72 -> [w286 _]
      tunnel: w71 -> [w285 _]
      tunnel: w69 -> [w279 _]
      tunnel: w68 -> [w278 _]
      tunnel: "Set VDD" -> [w277 _]
      tunnel: [w276 _] -> w64
      frame False {
        w316 = u64 0 ("Total Completed")
        w296 = u32 100 ("milliseconds to wait")
        w332 = T7 [enum."Voltage 2", enum."Voltage 3", enum."Voltage 1"] items=["Idle...", "Voltage 1", "Voltage 2", "Voltage 3"]
        w334 = T7 [enum."Voltage 2", enum."Voltage 3", enum."Voltage 1"] items=["Idle...", "Voltage 1", "Voltage 2", "Voltage 3"]
        # "VSA"
        # "HS"
        # "HD/CYC"
        # "DVA"
        # "E-CAL"
        # "VPI"
        # "Verify Socket"
        n89 = for {
          tunnel: w336 -> [w2002]
          tunnel: w335 -> [w2001]
          tunnel: w334 -> [w1999] mode=indexing
          tunnel: [w1995] -> w329
          tunnel: [w1998] -> w319
          tunnel: w277 -> [w1992]
          n90 = call "E3631A_Voltage Controller updated.vi"("VISA resource name"=w2001, "I_VDD(A)"=0.5, "Channel Controller"=w1999, "Voltage 1"=w1992, "Voltage 2"=3.3, "error in (no error)"=w2002, "I_3.3V (A)"=0.5) -> ("VISA resource name out"=w1998:refnum<visa-resource-name>, "error out"=w1996:errorcluster)  [unwired: 7 in]
          n91 = call "Delay.vi"("milliseconds to wait"=u32 100, "error in (no error)"=w1996) -> ("error out"=w1995:errorcluster)  [unwired: 9 in]
        }
        n92 = local write "TTCompleted"(w316) -> ()
        n93 = local write "Total Time"(w316) -> ()
        n94 = call "WSVCAP SHL Host TL RFFE Write - Multiple DUTs - Common Data.vi"("Data Out"="074000", "error in"=w329, "Log (T)"=FALSE) -> ("error out"=w330:errorcluster)  [unwired: 12 in]
        n95 = local read "IDD Brd(uA)"() -> (w304:string)
        n96 = call "Delay.vi"("milliseconds to wait"=w296, "error in (no error)"=w330) -> ("error out"=w328:errorcluster)  [unwired: 9 in]
        n97 = call "Ke2000 Single Reading.vi"("error in (no error)"=w328, "VISA resource name"=w327) -> ("error out"=w305:errorcluster, "VISA resource name out"=w326:refnum<visa-resource-name>, "uA"=w307:string)  [unwired: 5 in, 2 out]
        n98 = call "Substration.vi"("error in (no error)"=w305, "Input2"=w304, "Input1"=w307) -> ("error out"=w281:errorcluster, "In1 - In2"=w306:string)  [unwired: 7 in]
        "IDD Stdby(uA)" <- w306
        n99 = case shown="True" w290 {
          tunnel: [1 ("X Repeat") w409] -> w318
          frame False {
          }
          frame True {
            n100 = local read "X Repeat"() -> (w409:i32)
          }
        }
        n101 = call "WSVCAP SHL Host TL RFFE Write - Multiple DUTs - Common Data.vi"("Data Out"="074040", "error in"=w281, "Log (T)"=FALSE) -> ("error out"=w280:errorcluster)  [unwired: 12 in]
        n102 = call "Delay.vi"("milliseconds to wait"=w296, "error in (no error)"=w280) -> ("error out"=w313:errorcluster)  [unwired: 9 in]
        n103 = case shown="True" w288 {
          tunnel: w313 -> [w360 w369]
          tunnel: [w359 w367] -> w311
          tunnel: ["DVA OFF" ("Data Out") "DVA ON" ("Data Out")] -> w312
          frame False {
            n104 = call "WSVCAP SHL Host TL RFFE Write - Multiple DUTs - Common Data.vi"("Data Out"="074820", "error in"=w360) -> ("error out"=w359:errorcluster)  [unwired: 13 in]
          }
          frame True {
            n105 = call "WSVCAP SHL Host TL RFFE Write - Multiple DUTs - Common Data.vi"("Data Out"="074800", "error in"=w369, "Log (T)"=FALSE) -> ("error out"=w365:errorcluster)  [unwired: 12 in]
            n106 = case shown="1" "CP with DVA ON" {
              selector: "CP with DVA ON" -> [w375 w379 w383 w387 w391 w395 w399 w403 w407]
              tunnel: [w374 w378 w382 w386 w390 w394 w398 w402 w405] -> w362
              tunnel: [w373 w377 w381 w385 w389 w393 w397 w401 w406] -> w364
              tunnel: w365 -> [w373 w377 w381 w385 w389 w393 w397 w401 w406]
              tunnel: string[] ["07476F", "074776", "074765", "074769", "07477B", "07477C", "07477D", "074779", "07476B"] -> [w372 w376 w380 w384 w388 w392 w396 w400 w404]
              frame 0, Default {
                n107 = Index Array(array=w372, index=w375) -> (element=w374:string)
              }
              frame 2 {
                n108 = Index Array(array=w376, index=w379) -> (element=w378:string)
              }
              frame 3 {
                n109 = Index Array(array=w380, index=w383) -> (element=w382:string)
              }
              frame 4 {
                n110 = Index Array(array=w384, index=w387) -> (element=w386:string)
              }
              frame 5 {
                n111 = Index Array(array=w388, index=w391) -> (element=w390:string)
              }
              frame 6 {
                n112 = Index Array(array=w392, index=w395) -> (element=w394:string)
              }
              frame 7 {
                n113 = Index Array(array=w396, index=w399) -> (element=w398:string)
              }
              frame 8 {
                n114 = Index Array(array=w400, index=w403) -> (element=w402:string)
              }
              frame 1 {
                n115 = Index Array(array=w404, index=w407) -> (element=w405:string)
              }
            }
            n116 = call "WSVCAP SHL Host TL RFFE Write - Multiple DUTs - Common Data.vi"("Data Out"=w362, "error in"=w364, "Log (T)"=FALSE) -> ("error out"=w367:errorcluster)  [unwired: 12 in]
          }
        }
        n117 = for {
          N: 36 -> [_]
          tunnel: "Serial Number" -> [w342]
          tunnel: [w340] -> w293 mode=indexing
          i -> [w339]
          n118 = Increment(x=w339) -> (x+1=w338:i32)
          n119 = Index Array(array=w342, index (row)=w338, index (col)=1 ("disabled index (col)")) -> (element=w340:string)
        }
        n120 = Not(x=w285) -> (.not. x?=w292:bool)
        n121 = Number To Fractional String(number=w277, precision (6)=i16 2) -> (F-format string=w309:string)  [unwired: 2 in]
        n122 = call "Delay.vi"("milliseconds to wait"=w296, "error in (no error)"=w311) -> ("error out"=w299:errorcluster)  [unwired: 9 in]
        n123 = case shown="True" w289 {
          tunnel: w299 -> [w346 w348]
          tunnel: [w343 w347] -> w298
          tunnel: ["CAL OFF" ("Data Out") "CAL ON" ("Data Out")] -> w300
          frame False {
            n124 = call "WSVCAP SHL Host TL RFFE Write - Multiple DUTs - Common Data.vi"("Data Out"="074044", "error in"=w346) -> ("error out"=w343:errorcluster)  [unwired: 13 in]
          }
          frame True {
            n125 = for {
              tunnel: string[] ["074900", "074920", "074900"] -> [w356] mode=indexing
              tunnel: w348 -> [w353]
              tunnel: [w352] -> w347
              n126 = call "WSVCAP SHL Host TL RFFE Write - Multiple DUTs - Common Data.vi"("Data Out"=w356, "error in"=w353, "Log (T)"=FALSE) -> ("error out"=w355:errorcluster)  [unwired: 12 in]
              n127 = call "Delay.vi"("milliseconds to wait"=u32 10, "error in (no error)"=w355) -> ("error out"=w352:errorcluster)  [unwired: 9 in]
            }
          }
        }
        n128 = for {
          N: w318 -> [_]
          tunnel: w337 -> [w447]
          tunnel: [w443] -> w333
          tunnel: w306 -> [w442]
          tunnel: w326 -> [w441]
          tunnel: "TMN DC\\CAP Data Log File Path" -> [w440]
          tunnel: w324 -> [w438]
          tunnel: [w437] -> w322
          tunnel: w319 -> [w413]
          shift-right: [w432] -> _
          shift-left: u64 0 -> [w434]
          tunnel: w290 -> [w431]
          tunnel: w315 -> [w426]
          tunnel: w315 -> [w425]
          tunnel: w312 -> [w424]
          tunnel: w309 -> [w423]
          tunnel: [w422] -> w303
          tunnel: w300 -> [w421]
          tunnel: w298 -> [w420]
          tunnel: w288 -> [w419]
          tunnel: w291 -> [w418]
          tunnel: w287 -> [w417]
          tunnel: w292 -> [w416]
          tunnel: w286 -> [w415]
          tunnel: w293 -> [w414]
          tunnel: [w413] -> w282
          tunnel: w279 -> [w412]
          tunnel: w278 -> [w411]
          tunnel: [w410] -> w276
          i -> [w430]
          stop <- w410 stop-if-true
          n129 = while {
            tunnel: w447 -> [w668]
            tunnel: w440 -> [w679]
            tunnel: "Lot#" -> [w678]
            tunnel: "Wafer#" -> [w677]
            tunnel: w414 -> [w676]
            tunnel: "Test Program" -> [w675]
            tunnel: w414 -> [w674]
            tunnel: "Comment" -> [w673]
            tunnel: "Lot#" -> [w672]
            tunnel: "Wafer#" -> [w671]
            tunnel: w441 -> [w667]
            tunnel: [w670] -> w443
            tunnel: w442 -> [w666]
            tunnel: w438 -> [w663]
            tunnel: [w662] -> w437
            tunnel: [w570] -> w428
            tunnel: w430 -> [w608]
            tunnel: [w599] -> w432
            tunnel: w434 -> [w598]
            shift-right: [w597] -> _
            shift-left: u64 0 -> [w494]
            tunnel: [w596] -> w427
            tunnel: w431 -> [w594]
            tunnel: w426 -> [w569]
            tunnel: w425 -> [w567]
            tunnel: w424 -> [w517]
            tunnel: w423 -> [w515]
            tunnel: [w491] -> w422
            tunnel: w421 -> [w498]
            tunnel: w420 -> [w497]
            tunnel: w419 -> [w496]
            tunnel: w418 -> [w488]
            tunnel: w417 -> [w487]
            tunnel: w416 -> [w482]
            tunnel: w415 -> [w476]
            tunnel: w412 -> [w452]
            tunnel: w411 -> [w451]
            i -> [w595]
            stop <- w609 stop-if-true
            n130 = case shown="8" "CP to HD/Cycle" {
              selector: "CP to HD/Cycle" -> [w683 w688 w693 w698 w703 w708 w713 w718 w722]
              tunnel: string[] ["07476F", "074776", "074765", "074769", "07477B", "07477C", "07477D", "074779", "07476B"] -> [w684 w689 w694 w699 w704 w709 w714 w719 w724]
              tunnel: [w682 w687 w692 w697 w702 w707 w712 w717 w723] -> w513
              tunnel: ["35.0" ("Data Out") "27.5" ("Data Out") "30.5" ("Data Out") "44.0" ("Data Out") "50.0" ("Data Out") "55.0" ("Data Out") "42.5" ("Data Out") "32.0" ("Data Out") "40.25" ("Data Out")] -> w512
              tunnel: [w680 w685 w690 w695 w700 w705 w710 w715 w720] -> w511
              tunnel: w497 -> [w680 w685 w690 w695 w700 w705 w710 w715 w720]
              frame 0, Default {
                n131 = Index Array(array=w684, index=w683) -> (element=w682:string)
              }
              frame 2 {
                n132 = Index Array(array=w689, index=w688) -> (element=w687:string)
              }
              frame 3 {
                n133 = Index Array(array=w694, index=w693) -> (element=w692:string)
              }
              frame 4 {
                n134 = Index Array(array=w699, index=w698) -> (element=w697:string)
              }
              frame 5 {
                n135 = Index Array(array=w704, index=w703) -> (element=w702:string)
              }
              frame 6 {
                n136 = Index Array(array=w709, index=w708) -> (element=w707:string)
              }
              frame 7 {
                n137 = Index Array(array=w714, index=w713) -> (element=w712:string)
              }
              frame 8 {
                n138 = Index Array(array=w719, index=w718) -> (element=w717:string)
              }
              frame 1 {
                n139 = Index Array(array=w724, index=w722) -> (element=w723:string)
              }
            }
            n140 = flat-sequence {
              tunnel: [w792] -> w661
              tunnel: [w787] -> w660
              tunnel: w668 -> [w790]
              tunnel: [w789] -> w659
              tunnel: w667 -> [w767]
              tunnel: w666 -> [w788]
              tunnel: [w788] -> w658
              tunnel: [w740] -> w657
              tunnel: [w737] -> w656
              tunnel: w511 -> [w780]
              tunnel: w608 -> [w785]
              tunnel: w595 -> [w763]
              tunnel: [w763] -> w605
              tunnel: w595 -> [w784]
              tunnel: w594 -> [w782]
              tunnel: [w781] -> w593
              tunnel: [w746] -> w588
              tunnel: [w745] -> w587
              tunnel: [w744] -> w586
              tunnel: [w750] -> w576
              tunnel: [w747] -> w575
              tunnel: w569 -> [w779]
              tunnel: [w779] -> w568
              tunnel: w567 -> [w778]
              tunnel: [w749] -> w555
              tunnel: [w748] -> w530
              tunnel: [w777] -> w518
              tunnel: w513 -> [w775]
              tunnel: [w764] -> w510
              tunnel: [w730] -> w502
              tunnel: w488 -> [w760]
              tunnel: w487 -> [w759]
              tunnel: [w759] -> w486
              tunnel: w482 -> [w758]
              tunnel: [w758] -> w481
              tunnel: w476 -> [w757]
              tunnel: [w757] -> w475
              tunnel: [w753] -> w470
              tunnel: ["Test Sequences"] -> w466
              tunnel: "Real No. From\nLookup Table" -> [w743]
              tunnel: ["WS1050/51"] -> w460
              tunnel: ["Cmin/Act"] -> w456
              tunnel: w452 -> [w732]
              tunnel: w451 -> [w731]
              tunnel: w661 -> [w1101]
              tunnel: w660 -> [w1126]
              tunnel: w659 -> [w1131]
              tunnel: [w1131] -> w566
              tunnel: w658 -> [w1130]
              tunnel: w657 -> [w1125]
              tunnel: w656 -> [w1124]
              tunnel: [w1115] -> w565
              tunnel: [w1130] -> w564
              tunnel: [w1125] -> w563
              tunnel: [w1124] -> w562
              tunnel: w605 -> [w1128]
              tunnel: [w1128] -> w561
              tunnel: w593 -> [w1127]
              tunnel: [w1127] -> w560
              tunnel: [w1126] -> w559
              tunnel: w588 -> [w1123]
              tunnel: w587 -> [w1108]
              tunnel: w586 -> [w1109]
              tunnel: [w1120] -> w558
              tunnel: w576 -> [w1122]
              tunnel: w575 -> [w1120]
              tunnel: [w1116] -> w557
              tunnel: w568 -> [w1121]
              tunnel: [w1106] -> w556
              tunnel: w555 -> [w1106]
              tunnel: [w1108] -> w554
              tunnel: w530 -> [w1107]
              tunnel: [w1107] -> w529
              tunnel: [w1109] -> w527
              tunnel: w518 -> [w1119]
              tunnel: [w1118] -> w503
              tunnel: w502 -> [w1118]
              tunnel: w486 -> [w1114]
              tunnel: [w1114] -> w485
              tunnel: w481 -> [w1113]
              tunnel: [w1113] -> w480
              tunnel: w475 -> [w1112]
              tunnel: [w1112] -> w474
              tunnel: w470 -> [w1111]
              tunnel: [w1110] -> w469
              tunnel: w466 -> [w1104]
              tunnel: [w1104] -> w465
              tunnel: w460 -> [w1103]
              tunnel: [w1103] -> w459
              tunnel: w456 -> [w1102]
              tunnel: [w1102] -> w455
              tunnel: [w1101] -> w449
              tunnel: w566 -> [w1253]
              tunnel: [w1253] -> w551
              tunnel: w565 -> [w1235]
              tunnel: [w1235] -> w549
              tunnel: w564 -> [w1252]
              tunnel: [w1252] -> w547
              tunnel: w563 -> [w1251]
              tunnel: [w1251] -> w545
              tunnel: w562 -> [w1250]
              tunnel: [w1250] -> w543
              tunnel: w561 -> [w1249]
              tunnel: [w1249] -> w541
              tunnel: w560 -> [w1248]
              tunnel: [w1248] -> w539
              tunnel: w559 -> [w1247]
              tunnel: [w1247] -> w537
              tunnel: w558 -> [w1246]
              tunnel: [w1246] -> w535
              tunnel: [w1240] -> w533
              tunnel: w557 -> [w1239]
              tunnel: w556 -> [w1244]
              tunnel: w554 -> [w1243]
              tunnel: w529 -> [w1232]
              tunnel: [w1232] -> w528
              tunnel: w527 -> [w1234]
              tunnel: [w1234] -> w526
              tunnel: [w1241] -> w525
              tunnel: [w1242] -> w504
              tunnel: w503 -> [w1242]
              tunnel: w485 -> [w1238]
              tunnel: [w1238] -> w484
              tunnel: w480 -> [w1237]
              tunnel: [w1237] -> w479
              tunnel: w474 -> [w1236]
              tunnel: [w1236] -> w473
              tunnel: w469 -> [w1233]
              tunnel: w465 -> [w1230]
              tunnel: [w1233] -> w464
              tunnel: [w1230] -> w463
              tunnel: w459 -> [w1229]
              tunnel: [w1229] -> w458
              tunnel: w455 -> [w1228]
              tunnel: [w1228] -> w454
              tunnel: w449 -> [w1227]
              tunnel: [w1227] -> w448
              tunnel: [w1320] -> w553
              tunnel: [w1332] -> w552
              tunnel: w551 -> [w1347]
              tunnel: [w1347] -> w550
              tunnel: w549 -> [w1326]
              tunnel: [w1326] -> w548
              tunnel: w547 -> [w1346]
              tunnel: [w1346] -> w546
              tunnel: w545 -> [w1345]
              tunnel: [w1345] -> w544
              tunnel: w543 -> [w1344]
              tunnel: [w1344] -> w542
              tunnel: w541 -> [w1343]
              tunnel: [w1343] -> w540
              tunnel: w539 -> [w1342]
              tunnel: [w1342] -> w538
              tunnel: w537 -> [w1341]
              tunnel: [w1341] -> w536
              tunnel: w535 -> [w1340]
              tunnel: [w1340] -> w534
              tunnel: w533 -> [w1339]
              tunnel: [w1339] -> w532
              tunnel: [w1323] -> w531
              tunnel: w528 -> [w1337]
              tunnel: w526 -> [w1336]
              tunnel: w525 -> [w1331]
              tunnel: ["DeltaC Target Setting(pF)"] -> w516
              tunnel: [w1334] -> w505
              tunnel: w504 -> [w1334]
              tunnel: w496 -> [w1333]
              tunnel: [w1333] -> w495
              tunnel: w484 -> [w1330]
              tunnel: [w1330] -> w483
              tunnel: w479 -> [w1329]
              tunnel: [w1329] -> w478
              tunnel: w473 -> [w1328]
              tunnel: [w1328] -> w472
              tunnel: w464 -> [w1327]
              tunnel: w463 -> [w1324]
              tunnel: [w1323] -> w461
              tunnel: w458 -> [w1322]
              tunnel: [w1322] -> w457
              tunnel: w454 -> [w1321]
              tunnel: [w1321] -> w453
              tunnel: w448 -> [w1320]
              tunnel: [w1414] -> w655
              tunnel: [w1434] -> w654
              tunnel: w553 -> [w1414]
              tunnel: w552 -> [w1448]
              tunnel: [w1457] -> w653
              tunnel: [w1448] -> w652
              tunnel: [w1470] -> w651
              tunnel: [w1469] -> w650
              tunnel: w550 -> [w1468]
              tunnel: [w1468] -> w649
              tunnel: w548 -> [w1457]
              tunnel: w546 -> [w1467]
              tunnel: [w1467] -> w648
              tunnel: w544 -> [w1463]
              tunnel: [w1463] -> w647
              tunnel: w542 -> [w1462]
              tunnel: [w1462] -> w646
              tunnel: w540 -> [w1458]
              tunnel: [w1458] -> w604
              tunnel: w538 -> [w1466]
              tunnel: [w1466] -> w592
              tunnel: w536 -> [w1465]
              tunnel: [w1464] -> w589
              tunnel: w534 -> [w1460]
              tunnel: w532 -> [w1456]
              tunnel: [w1461] -> w585
              tunnel: [w1459] -> w584
              tunnel: [w1456] -> w579
              tunnel: w531 -> [w1455]
              tunnel: [w1442] -> w574
              tunnel: [w1441] -> w573
              tunnel: [w1440] -> w572
              tunnel: w516 -> [w1454]
              tunnel: [w1439] -> w506
              tunnel: w505 -> [w1439]
              tunnel: [w1438] -> w501
              tunnel: w495 -> [w1437]
              tunnel: w483 -> [w1432]
              tunnel: w478 -> [w1431]
              tunnel: [w1431] -> w477
              tunnel: w472 -> [w1430]
              tunnel: [w1430] -> w471
              tunnel: w461 -> [w1427]
              tunnel: w457 -> [w1426]
              tunnel: w453 -> [w1415]
              tunnel: w655 -> [w1665]
              tunnel: [w1665] -> w645
              tunnel: [w1692] -> w644
              tunnel: [w1706] -> w643
              tunnel: w654 -> [w1705]
              tunnel: w653 -> [w1704]
              tunnel: w652 -> [w1703]
              tunnel: [w1704] -> w642
              tunnel: [w1703] -> w641
              tunnel: w651 -> [w1702]
              tunnel: [w1702] -> w640
              tunnel: w650 -> [w1701]
              tunnel: [w1701] -> w639
              tunnel: w649 -> [w1700]
              tunnel: [w1700] -> w638
              tunnel: w648 -> [w1699]
              tunnel: [w1699] -> w637
              tunnel: w647 -> [w1698]
              tunnel: [w1698] -> w636
              tunnel: w646 -> [w1697]
              tunnel: [w1697] -> w635
              tunnel: w663 -> [w1696]
              tunnel: [w1694] -> w634
              tunnel: [w1674] -> w633
              tunnel: [w1675] -> w632
              tunnel: [w1673] -> w631
              tunnel: w604 -> [w1690]
              tunnel: [w1690] -> w603
              tunnel: w592 -> [w1689]
              tunnel: [w1689] -> w591
              tunnel: w589 -> [w1706]
              tunnel: w585 -> [w1687]
              tunnel: w584 -> [w1688]
              tunnel: [w1688] -> w583
              tunnel: [w1687] -> w581
              tunnel: w579 -> [w1686]
              tunnel: [w1686] -> w578
              tunnel: w574 -> [w1672]
              tunnel: w573 -> [w1671]
              tunnel: w572 -> [w1670]
              tunnel: [w1667] -> w571
              tunnel: [w1672] -> w524
              tunnel: [w1671] -> w522
              tunnel: [w1670] -> w520
              tunnel: [w1669] -> w507
              tunnel: w506 -> [w1669]
              tunnel: w501 -> [w1668]
              tunnel: [w1668] -> w500
              tunnel: w477 -> [w1667]
              tunnel: w471 -> [w1666]
              tunnel: w645 -> [w1814]
              tunnel: [w1814] -> w630
              tunnel: w644 -> [w1838]
              tunnel: [w1837] -> w629
              tunnel: w679 -> [w1839]
              tunnel: w678 -> [w1836]
              tunnel: w677 -> [w1835]
              tunnel: w676 -> [w1834]
              tunnel: [w1833] -> w628
              tunnel: w643 -> [w1827]
              tunnel: [w1827] -> w627
              tunnel: w642 -> [w1832]
              tunnel: w641 -> [w1831]
              tunnel: [w1832] -> w626
              tunnel: [w1831] -> w625
              tunnel: [w1822] -> w624
              tunnel: w640 -> [w1830]
              tunnel: [w1830] -> w623
              tunnel: w639 -> [w1829]
              tunnel: [w1829] -> w622
              tunnel: w638 -> [w1826]
              tunnel: [w1828] -> w621
              tunnel: w494 -> [w1825]
              tunnel: [w1824] -> w620
              tunnel: [w1812] -> w619
              tunnel: w637 -> [w1823]
              tunnel: w636 -> [w1821]
              tunnel: w635 -> [w1820]
              tunnel: "File Name" -> [w1819]
              tunnel: w634 -> [w1818]
              tunnel: [w1818] -> w618
              tunnel: w633 -> [w1817]
              tunnel: [w1817] -> w617
              tunnel: [w1816] -> w616
              tunnel: w632 -> [w1816]
              tunnel: w631 -> [w1815]
              tunnel: [w1815] -> w615
              tunnel: [w1810] -> w606
              tunnel: w603 -> [w1811]
              tunnel: [w1811] -> w601
              tunnel: w598 -> [w1809]
              tunnel: w591 -> [w1808]
              tunnel: [w1808] -> w590
              tunnel: w583 -> [w1807]
              tunnel: [w1807] -> w582
              tunnel: w581 -> [w1806]
              tunnel: [w1806] -> w580
              tunnel: w578 -> [w1805]
              tunnel: [w1805] -> w577
              tunnel: w571 -> [w1804]
              tunnel: w524 -> [w1803]
              tunnel: [w1803] -> w523
              tunnel: w522 -> [w1802]
              tunnel: [w1802] -> w521
              tunnel: w520 -> [w1801]
              tunnel: [w1801] -> w519
              tunnel: w510 -> [w1800]
              tunnel: [w1800] -> w509
              tunnel: [w1799] -> w508
              tunnel: w507 -> [w1799]
              tunnel: w500 -> [w1798]
              tunnel: [w1798] -> w499
              tunnel: ["Freq(Hz)"] -> w468
              tunnel: ["Board#"] -> w467
              tunnel: w630 -> [w1860]
              tunnel: w629 -> [w1911]
              tunnel: w679 -> [w1875]
              tunnel: w675 -> [w1906]
              tunnel: w674 -> [w1909]
              tunnel: w673 -> [w1905]
              tunnel: w672 -> [w1908]
              tunnel: w671 -> [w1904]
              tunnel: w628 -> [w1907]
              tunnel: [w1860] -> w611
              tunnel: [w1910] -> w612
              tunnel: w627 -> [w1903]
              tunnel: [w1903] -> w613
              tunnel: w626 -> [w1902]
              tunnel: w625 -> [w1887]
              tunnel: w624 -> [w1901]
              tunnel: w623 -> [w1900]
              tunnel: w622 -> [w1889]
              tunnel: [w1897] -> w614
              tunnel: w621 -> [w1899]
              tunnel: w620 -> [w1898]
              tunnel: w619 -> [w1897]
              tunnel: "File Name" -> [w1868]
              tunnel: w618 -> [w1896]
              tunnel: [w1896] -> w610
              tunnel: w617 -> [w1895]
              tunnel: w616 -> [w1894]
              tunnel: w615 -> [w1893]
              tunnel: [w1892] -> w607
              tunnel: w606 -> [w1892]
              tunnel: [w1871] -> w602
              tunnel: w601 -> [w1871]
              tunnel: w590 -> [w1891]
              tunnel: w582 -> [w1890]
              tunnel: w580 -> [w1888]
              tunnel: w577 -> [w1886]
              tunnel: w523 -> [w1885]
              tunnel: w521 -> [w1884]
              tunnel: w519 -> [w1883]
              tunnel: w517 -> [w1882]
              tunnel: w498 -> [w1881]
              tunnel: w512 -> [w1880]
              tunnel: w515 -> [w1879]
              tunnel: w509 -> [w1878]
              tunnel: w508 -> [w1877]
              tunnel: w499 -> [w1876]
              tunnel: [w1873] -> w493
              tunnel: [w1864] -> w489
              tunnel: w468 -> [w1863]
              tunnel: w467 -> [w1861]
              tunnel: [w1961] -> w669
              tunnel: [w1962] -> w670
              tunnel: [w1963] -> w570
              tunnel: w614 -> [w1954]
              tunnel: w613 -> [w1962]
              tunnel: w612 -> [w1950]
              tunnel: w611 -> [w1963]
              tunnel: w610 -> [w1956]
              tunnel: [w1956] -> w662
              tunnel: [w1953] -> w599
              tunnel: w607 -> [w1953]
              tunnel: w602 -> [w1955]
              tunnel: [w1955] -> w600
              tunnel: [w1954] -> w597
              tunnel: [w1952] -> w596
              tunnel: [w1949] -> w490
              tunnel: w493 -> [w1948]
              tunnel: w489 -> [w1946]
              frame #0 {
                w754 = FALSE ("Log (T)")
                n141 = call "WSVCAP SHL Host TL RFFE Write - Multiple DUTs - Common Data.vi"("Data Out"=w775, "error in"=w780, "Log (T)"=FALSE) -> ("error out"=w761:errorcluster)  [unwired: 12 in]
                n142 = Index Array(array=w790, index (row)=w784, index (col)=0 ("disabled index (col)")) -> (element=w783:dbl)
                n143 = for {
                  tunnel: string[] ["0760", "0767", "0768"] -> [w859] mode=indexing
                  tunnel: [w855] -> w765 mode=indexing
                  tunnel: w761 -> [w853]
                  tunnel: [w852] -> w762
                  i -> [w858]
                  n144 = call "Delay.vi"("milliseconds to wait"=u32 10, "error in (no error)"=w853) -> ("error out"=w860:errorcluster)  [unwired: 9 in]
                  n145 = call "WSVCAP SHL Host TL RFFE Read - Multiple DUTs - Common Data.vi"("Data Out"=w859, "error in"=w860, "Log (T)"=FALSE) -> ("RFFE Data In"=w857:string[], "error out"=w852:errorcluster)  [unwired: 11 in]
                  n146 = Index Array(array=w857, index=w858) -> (element=w854:string)
                  n147 = String Subset(string=w854, offset (0)=0) -> (substring=w855:string)  [unwired: 1 in]
                }
                "RB Reg for HD/Cycle" <- w765
                n148 = local read "IDD Brd(uA)"() -> (w774:string)
                n149 = call "Delay.vi"("milliseconds to wait"=u32 100, "error in (no error)"=w762) -> ("error out"=w770:errorcluster)  [unwired: 9 in]
                n150 = call "Ke2000 Single Reading.vi"("error in (no error)"=w770, "VISA resource name"=w767) -> ("error out"=w772:errorcluster, "VISA resource name out"=w742:refnum<visa-resource-name>, "uA"=w773:string)  [unwired: 5 in, 2 out]
                n151 = call "Substration.vi"("error in (no error)"=w772, "Input2"=w774, "Input1"=w773) -> ("error out"=w769:errorcluster, "In1 - In2"=→"IDD_HD/CYC (uA)":string)  [unwired: 7 in]
                n152 = case shown="True" w782 {
                  tunnel: [w891 w996] -> w792
                  tunnel: [w892 w981] -> w728
                  tunnel: [w890 w997] -> w789
                  tunnel: w769 -> [w886 w985]
                  tunnel: w785 -> [_ w987]
                  tunnel: w783 -> [w883 w982]
                  tunnel: [w888 w983] -> w781
                  tunnel: w763 -> [w875 w979]
                  tunnel: w778 -> [w885 _]
                  tunnel: ["% Duty Cycle" "100" ("Data Out")] -> w764
                  tunnel: w760 -> [w873 _]
                  tunnel: w743 -> [w872 w974]
                  tunnel: w732 -> [w869 _]
                  tunnel: w731 -> [w868 _]
                  frame False {
                    # "Cycles in 1s"
                    n153 = case shown="True" w872 {
                      tunnel: w886 -> [w898 w904]
                      tunnel: w883 -> [w897 w903]
                      tunnel: [w896 w904] -> w882
                      tunnel: w875 -> [w895 _]
                      tunnel: [w894 w903] -> w881
                      tunnel: [u64 1000 ("y") u64 1 ("y")] -> w876
                      frame False {
                        n154 = case shown="8, Default" w895 {
                          tunnel: w897 -> [w900 _]
                          tunnel: [w900 "Cycle RP"] -> w894
                          tunnel: [w899 w901] -> w896
                          tunnel: w898 -> [w899 w901]
                          frame 0..7 {
                          }
                          frame 8, Default {
                          }
                        }
                      }
                      frame True {
                        # "Read real number\nfrom lookup table"
                      }
                    }
                    n155 = call "WSVCAP SHL Host TL RFFE Configure.vi"("RFFE Slave Address"=w885, "Clock Rate (Hz)"="SPI Clock Rate (Hz)", "error in"=w882) -> ("Actual Rate (Hz)"=→"AR Cycling(Hz)":dbl, "error out"=w871:errorcluster)  [unwired: 11 in]
                    n156 = Array Max & Min(array=w868) -> (max value=w879:dbl)  [unwired: 3 out]
                    n157 = Divide(x=1.0, y=w879) -> (x/y=w878:dbl)
                    n158 = To Unsigned Quad Integer(1:w878) -> (0:w877:u64)
                    n159 = Not(x=w873) -> (.not. x?=w874:bool)
                    n160 = case shown="True" w874 {
                      tunnel: [w907 w929] -> w892
                      tunnel: [w910 w928] -> w891
                      tunnel: [u64 1 w927] -> w890
                      tunnel: w871 -> [w908 w926]
                      tunnel: w881 -> [_ w925]
                      tunnel: w868 -> [_ w923]
                      tunnel: w877 -> [_ w922]
                      tunnel: w876 -> [_ w921]
                      tunnel: w875 -> [w906 _]
                      tunnel: w869 -> [_ w920]
                      frame False {
                        n161 = case shown="1, Default" w906 {
                          tunnel: w908 -> [w911 w913]
                          tunnel: [w911 w912] -> w907
                          frame 0 {
                          }
                          frame 1, Default {
                            n162 = flat-sequence {
                              tunnel: "Repeat Meas(s)" -> [w919]
                              tunnel: w913 -> [w916]
                              tunnel: [w916] -> w912
                              frame #0 {
                                n163 = Multiply(x=w919, y=u32 1000) -> (x*y=w918:u32)
                                n164 = Wait (ms)(milliseconds to wait=w918) -> ()  [unwired: 1 out]
                                n165 = local write "STATUS"("Verify Sockets waiting times..." ("STATUS")) -> ()
                              }
                            }
                          }
                        }
                        n166 = local read "stop During HD/Cycles"() -> (w910:bool)
                      }
                      frame True {
                        n167 = while {
                          tunnel: w925 -> [w949]
                          tunnel: [w936] -> w929
                          tunnel: [w941] -> w928
                          tunnel: w926 -> [w947]
                          tunnel: [w935] -> w927
                          tunnel: w920 -> [w946]
                          tunnel: w923 -> [w945]
                          tunnel: w922 -> [w932]
                          tunnel: w921 -> [w930]
                          i -> [w944]
                          stop <- w940 stop-if-true
                          # "At least 1 second before target"
                          # "Remaining Cycles"
                          # "Target Cycles"
                          # "Cycles in 1s"
                          n168 = To Unsigned Quad Integer(1:w949) -> (0:w948:u64)
                          n169 = case shown="0" w944 {
                            tunnel: [w957 w959] -> w938
                            tunnel: w947 -> [w958 w959]
                            tunnel: w946 -> [w956 _]
                            tunnel: w945 -> [w955 _]
                            frame 0 {
                              n170 = call "WSVCAP SHL Host TL RFFE Write Cycle - Multiple DUTs - Common Data.vi"("Data Out (Cycle Commands)"=w956, "Post Command Delay"=w955, "error in"=w958, "Log (T)"=FALSE) -> ("error out"=w957:errorcluster)  [unwired: 11 in]
                            }
                            frame 1, Default {
                            }
                          }
                          n171 = Multiply(x=w948, y=w930) -> (x*y=w935:u64)
                          n172 = call "WSVCAP SHL Host TL SPI_RFFE Query Cycle Count.vi"("error in"=w938) -> ("Cycle Count"=w934:u64, "error out"=w943:errorcluster)  [unwired: 13 in]
                          "Cycle Count" <- w934
                          n173 = Subtract(x=w935, y=w934) -> (x-y=w933:u64)
                          n174 = Greater Or Equal?(x=w934, y=w935) -> (x >= y?=w942:bool)
                          n175 = local read "stop During HD/Cycles"() -> (w941:bool)
                          n176 = Greater?(x=w933, y=w932) -> (0:w931:bool)
                          n177 = case shown="True" w942 {
                            tunnel: [w961 w964] -> w937
                            tunnel: w943 -> [w961 w963]
                            tunnel: [FALSE TRUE] -> w939
                            frame False {
                            }
                            frame True {
                              n178 = call "WSVCAP SHL Host TL SPI Stop Write Cycle.vi"("error in"=w963) -> ("error out"=w964:errorcluster)  [unwired: 14 in]
                            }
                          }
                          n179 = Or(x=w939, y=w941) -> (x .or. y?=w940:bool)
                          n180 = case shown="True" w931 {
                            tunnel: w937 -> [w950 w953]
                            tunnel: [w950 w952] -> w936
                            frame False {
                            }
                            frame True {
                              n181 = call "MISC Wait with Data Flow.vi"("Error In (no error)"=w953, "Wait Time (500ms)"=u32 50) -> ("Error Out"=w952:errorcluster)  [unwired: 7 in, 2 out]
                            }
                          }
                        }
                        n182 = local write "STATUS"("Parts are Cycling...." ("STATUS")) -> ()
                      }
                    }
                    n183 = local read "HD/CYC Temp"() -> (w887:i32)
                    n184 = Number To Engineering String(4:w887) -> (0:w888:string)  [unwired: 3 in]
                  }
                  frame True {
                    n185 = case shown="False" w974 {
                      tunnel: w987 -> [w1014 _]
                      tunnel: [w1013 w1026] -> w986
                      tunnel: w985 -> [w1012 w1027]
                      tunnel: [w1011 w1027] -> w984
                      tunnel: w982 -> [w1010 w1026]
                      tunnel: w979 -> [w1009 _]
                      frame False {
                        n186 = case shown="1, Default" w1014 {
                          tunnel: [w1017 w1024] -> w1013
                          tunnel: w1012 -> [w1019 w1025]
                          tunnel: [w1018 w1025] -> w1011
                          tunnel: w1010 -> [w1016 _]
                          tunnel: w1009 -> [w1015 _]
                          frame 0 {
                            n187 = case shown="15, Default" w1015 {
                              tunnel: [w1020 "HD RP"] -> w1017
                              tunnel: w1019 -> [w1021 w1022]
                              tunnel: [w1021 w1022] -> w1018
                              tunnel: w1016 -> [w1020 _]
                              frame 0..14 {
                              }
                              frame 15, Default {
                              }
                            }
                          }
                          frame 1, Default {
                            n188 = local read "HD RP"() -> (w1024:dbl)
                          }
                        }
                      }
                      frame True {
                      }
                    }
                    n189 = call "WSVCAP SHL Host TL RFFE Write - Multiple DUTs - Common Data.vi"("Data Out"="Cmd To HD", "error in"=w984, "Log (T)"=FALSE) -> ("error out"=w970:errorcluster)  [unwired: 12 in]
                    n190 = local read "No of HD/Cycle\nCompleted"() -> (w988:u64)
                    n191 = call "Delay.vi"("milliseconds to wait"=u32 50, "error in (no error)"=w970) -> ("error out"=w967:errorcluster)  [unwired: 9 in]
                    n192 = for {
                      tunnel: string[] ["0761", "0762", "0763"] -> [w1008] mode=indexing
                      tunnel: [w1004] -> w966 mode=indexing
                      shift-right: [w1001] -> w992
                      shift-left: w967 -> [w1007]
                      i -> [w1006]
                      n193 = call "WSVCAP SHL Host TL RFFE Read - Multiple DUTs - Common Data.vi"("Data Out"=w1008, "error in"=w1007, "Log (T)"=FALSE) -> ("RFFE Data In"=w1003:string[], "error out"=w1000:errorcluster)  [unwired: 11 in]
                      n194 = Index Array(array=w1003, index=w1006) -> (element=w1002:string)
                      n195 = call "Delay.vi"("milliseconds to wait"=u32 10, "error in (no error)"=w1000) -> ("error out"=w1001:errorcluster)  [unwired: 9 in]
                      n196 = String Subset(string=w1002, offset (0)=0) -> (substring=w1004:string)  [unwired: 1 in]
                    }
                    "RB Reg for HD" <- w966
                    n197 = Greater?(x="HD_DC (Min)", y=w988) -> (0:w989:bool)
                    n198 = case shown="True" w989 {
                      tunnel: [_ w1038] -> w994
                      tunnel: [w1029 w1037] -> w993
                      tunnel: w992 -> [w1029 w1036]
                      tunnel: w986 -> [w1028 w1035]
                      tunnel: [w1028 w1035] -> w991
                      frame False {
                      }
                      frame True {
                        n199 = Multiply(x=1000.0, y=w1035) -> (x*y=w1033:dbl)
                        n200 = Multiply(x=60.0, y=w1033) -> (x*y=w1031:dbl)
                        n201 = local write "STATUS"("Parts are Holding Down..." ("STATUS")) -> ()
                        n202 = event shown="[0] Timeout" {
                          selector: _ -> [_ _]
                          dyn-events: _ -> [_ _]
                          timeout: w1031 -> [_ _]
                          tunnel: ["stop During HD/Cycles" TRUE ("stop During HD/Cycles")] -> w1038
                          tunnel: w1036 -> [w1039 w1041]
                          tunnel: [w1039 w1041] -> w1037
                          event Timeout {
                            n203 = event-data() -> ()  [unwired: 1 in, 2 out]
                          }
                          event "stop During HD/Cycles": Value Change {
                            n204 = event-data() -> ()  [unwired: 1 in, 2 out]
                          }
                        }
                      }
                    }
                    n205 = Greater Or Equal?(x=w988, y="HD_DC (Min)") -> (x >= y?=w995:bool)
                    n206 = To Unsigned Quad Integer(1:w986) -> (0:w997:u64)
                    n207 = Add(x="Time All OFF (s)", y="Time All ON (s)") -> (x+y=w976:u32)
                    n208 = To Double Precision Float(number=w976) -> (double precision float=w975:dbl)
                    n209 = Divide(x=w975, y=60.0) -> (x/y=w977:dbl)
                    n210 = case shown="False" w995 {
                      tunnel: [w1045 w1061] -> w996
                      tunnel: [w1046 w1053] -> w981
                      tunnel: w993 -> [w1046 w1060]
                      tunnel: w994 -> [w1045 w1059]
                      tunnel: w991 -> [_ w1058]
                      tunnel: [w1044 w1056] -> w983
                      tunnel: w977 -> [_ w1050]
                      tunnel: "Time All OFF (s)" -> [_ w1048]
                      tunnel: "Time All ON (s)" -> [_ w1047]
                      frame False {
                        n211 = Number To Engineering String(4:"HD/CYC Temp") -> (0:w1044:string)  [unwired: 3 in]
                      }
                      frame True {
                        n212 = Divide(x=w1058, y=w1050) -> (x/y=w1057:dbl)
                        n213 = call "WSVCAP SHL Host TL RFFE Write - Multiple DUTs - Common Data.vi"("Data Out"="070201000000", "error in"=w1060, "Log (T)"=FALSE) -> ("error out"=w1063:errorcluster)  [unwired: 12 in]
                        n214 = Round To Nearest(number=w1057) -> (nearest integer value=w1052:dbl)
                        n215 = call "Delay.vi"("milliseconds to wait"=u32 50, "error in (no error)"=w1063) -> ("error out"=w1054:errorcluster)  [unwired: 9 in]
                        n216 = To Long Integer(number=w1052) -> (32bit integer=w1051:i32)
                        "No LPs to RP" <- w1051
                        n217 = for {
                          N: w1051 -> [_]
                          tunnel: w1059 -> [w1081]
                          tunnel: [w1080] -> w1061
                          tunnel: w1054 -> [w1070]
                          tunnel: [w1069] -> w1053
                          tunnel: w1048 -> [w1067]
                          tunnel: w1047 -> [w1065]
                          i -> [w1079]
                          stop <- w1080 stop-if-true
                          w1068 = FALSE ("Log (T)")
                          w1066 = u32 1 ("milliseconds to wait")
                          n218 = Increment(x=w1079) -> (x+1=→"LPs Count":i32)
                          n219 = call "WSVCAP SHL Host TL RFFE Write - Multiple DUTs - Common Data.vi"("Data Out"="074776", "error in"=w1070, "Log (T)"=w1068) -> ("error out"=w1087:errorcluster)  [unwired: 12 in]
                          n220 = call "Delay.vi"("milliseconds to wait"=w1066, "error in (no error)"=w1087) -> ("error out"=w1086:errorcluster)  [unwired: 9 in]
                          n221 = local read "CP to HD/Cycle"() -> (w1072:i32)
                          n222 = call "WSVCAP SHL Host TL RFFE Write - Multiple DUTs - Common Data.vi"("Data Out"="070201000000", "error in"=w1073) -> ("error out"=w1083:errorcluster)  [unwired: 13 in]
                          n223 = call "WSVCAP SHL Host TL RFFE Write - Multiple DUTs - Common Data.vi"("Data Out"="0702013B3B3B", "error in"=w1086, "Log (T)"=w1068) -> ("error out"=w1076:errorcluster)  [unwired: 12 in]
                          n224 = call "Delay.vi"("milliseconds to wait"=w1066, "error in (no error)"=w1076) -> ("error out"=w1075:errorcluster)  [unwired: 9 in]
                          n225 = flat-sequence {
                            tunnel: w1083 -> [w1094]
                            tunnel: [w1092] -> w1069
                            tunnel: w1067 -> [w1089]
                            frame #0 {
                              n226 = local write "STATUS"("Now HD OFF Time..." ("STATUS")) -> ()
                              n227 = Multiply(x=w1089, y=u32 1000) -> (x*y=w1091:u32)
                              n228 = call "Delay.vi"("milliseconds to wait"=w1091, "error in (no error)"=w1094) -> ("error out"=w1092:errorcluster)  [unwired: 9 in]
                            }
                          }
                          n229 = Index Array(array=string[] ["07476F", "074776", "074765", "074769", "07477B"], index=w1072) -> (element=w1077:string)
                          n230 = call "WSVCAP SHL Host TL RFFE Write - Multiple DUTs - Common Data.vi"("Data Out"=w1077, "error in"=w1075, "Log (T)"=w1068) -> ("error out"=w1074:errorcluster)  [unwired: 12 in]
                          n231 = flat-sequence {
                            tunnel: [w1099] -> w1073
                            tunnel: w1074 -> [w1096]
                            tunnel: w1065 -> [w1095]
                            frame #0 {
                              n232 = local write "STATUS"("Now HD ON Time..." ("STATUS")) -> ()
                              n233 = Multiply(x=w1095, y=u32 1000) -> (x*y=w1098:u32)
                              n234 = call "Delay.vi"("milliseconds to wait"=w1098, "error in (no error)"=w1096) -> ("error out"=w1099:errorcluster)  [unwired: 9 in]
                            }
                          }
                          n235 = Unbundle By Name(w1069) -> ("status"=w1082:bool)
                          n236 = Or(x=w1082, y=w1081) -> (x .or. y?=w1080:bool)
                        }
                        n237 = Number To Engineering String(4:"DC_Temp") -> (0:w1056:string)  [unwired: 3 in]
                      }
                    }
                  }
                }
                n238 = case shown="0, Default" "CP to Meas" {
                  selector: "CP to Meas" -> [w796 w801 w806 w811 w816 w821 w826 w831 w835]
                  tunnel: string[] ["07476F", "074776", "074765", "074769", "07477B", "07477C", "07477D", "074779", "07476B"] -> [w797 w802 w807 w812 w817 w822 w827 w832 w837]
                  tunnel: [w795 w800 w805 w810 w815 w820 w825 w830 w836] -> w726
                  tunnel: ["35.0" ("Data Out") "27.5" ("Data Out") "30.5" ("Data Out") "44.0" ("Data Out") "50.0" ("Data Out") "55.0" ("Data Out") "42.5" ("Data Out") "32.0" ("Data Out") "40.25" ("Data Out")] -> w730
                  tunnel: [w793 w798 w803 w808 w813 w818 w823 w828 w833] -> w729
                  tunnel: w728 -> [w793 w798 w803 w808 w813 w818 w823 w828 w833]
                  frame 0, Default {
                    n239 = Index Array(array=w797, index=w796) -> (element=w795:string)
                  }
                  frame 2 {
                    n240 = Index Array(array=w802, index=w801) -> (element=w800:string)
                  }
                  frame 3 {
                    n241 = Index Array(array=w807, index=w806) -> (element=w805:string)
                  }
                  frame 4 {
                    n242 = Index Array(array=w812, index=w811) -> (element=w810:string)
                  }
                  frame 5 {
                    n243 = Index Array(array=w817, index=w816) -> (element=w815:string)
                  }
                  frame 6 {
                    n244 = Index Array(array=w822, index=w821) -> (element=w820:string)
                  }
                  frame 7 {
                    n245 = Index Array(array=w827, index=w826) -> (element=w825:string)
                  }
                  frame 8 {
                    n246 = Index Array(array=w832, index=w831) -> (element=w830:string)
                  }
                  frame 1 {
                    n247 = Index Array(array=w837, index=w835) -> (element=w836:string)
                  }
                }
                n248 = call "WSVCAP SHL Host TL RFFE Write - Multiple DUTs - Common Data.vi"("Data Out"=w726, "error in"=w729, "Log (T)"=w754) -> ("error out"=w776:errorcluster)  [unwired: 12 in]
                n249 = flat-sequence {
                  tunnel: w756 -> [w862]
                  tunnel: [w862] -> w752
                  frame #0 {
                    w864 = "0" ("NOM IDD OFF(uA)")
                    w865 = string[] []
                    w866 = string[][] []
                    n250 = To Long Integer(number=0.0 ("No of Loops to RP")) -> (32bit integer=w863:i32)
                    n251 = local write "NOM IDD ON (uA)"(w864) -> ()
                    n252 = local write "NOM IDD OFF(uA)"(w864) -> ()
                    n253 = local write "LPs Count"(w863) -> ()
                    n254 = local write "No LPs to RP"(w863) -> ()
                    n255 = local write "Total Delta C1(pF)"(w865) -> ()
                    n256 = local write "Total Delta C2(pF)"(w865) -> ()
                    n257 = local write "Total Delta C3(pF)"(w865) -> ()
                    n258 = local write "Current EFuse Read back"(w865) -> ()
                    n259 = local write "RB Reg for HD"(w865) -> ()
                    n260 = local write "RB Reg for HD/Cycle"(w865) -> ()
                    n261 = local write "CAP_C3"(w866) -> ()
                    n262 = local write "CAP_C2"(w866) -> ()
                    n263 = local write "CAP_C1"(w866) -> ()
                    n264 = local write "VSA_V3"(w866) -> ()
                    n265 = local write "VSA_V1"(w866) -> ()
                    n266 = local write "VSA_V2"(w866) -> ()
                    n267 = local write "VPI C1"(w866) -> ()
                    n268 = local write "VPI C2"(w866) -> ()
                    n269 = local write "VPI C3"(w866) -> ()
                    n270 = local write "% Delta C"(w866) -> ()
                  }
                }
                n271 = call "Delay.vi"("milliseconds to wait"=u32 50, "error in (no error)"=w776) -> ("error out"=w735:errorcluster)  [unwired: 9 in]
                n272 = for {
                  tunnel: [w850] -> w787
                  tunnel: [w849] -> w756
                  tunnel: w754 -> [w848]
                  tunnel: w742 -> [w847]
                  tunnel: w735 -> [w843]
                  tunnel: string[] ["0702013B3B3B", "070201000000"] -> [w839] mode=indexing
                  tunnel: [w838] -> w738 mode=indexing
                  n273 = call "WSVCAP SHL Host TL RFFE Write - Multiple DUTs - Common Data.vi"("Data Out"=w839, "error in"=w843, "Log (T)"=w848) -> ("error out"=w844:errorcluster)  [unwired: 12 in]
                  n274 = local read "IDD Brd(uA)"() -> (w840:string)
                  n275 = call "Delay.vi"("milliseconds to wait"=u32 100, "error in (no error)"=w844) -> ("error out"=w845:errorcluster)  [unwired: 9 in]
                  n276 = call "Ke2000 Single Reading.vi"("error in (no error)"=w845, "VISA resource name"=w847) -> ("error out"=w842:errorcluster, "VISA resource name out"=w850:refnum<visa-resource-name>, "uA"=w841:string)  [unwired: 5 in, 2 out]
                  n277 = call "Substration.vi"("error in (no error)"=w842, "Input2"=w840, "Input1"=w841) -> ("error out"=w849:errorcluster, "In1 - In2"=w838:string)  [unwired: 7 in]
                }
                n278 = Index Array(array=w738, index=1) -> (element=w737:string)
                n279 = Index Array(array=w738, index=0) -> (element=w740:string)
                n280 = local read "Clock Rate (Hz)"() -> (w777:dbl)
                n281 = call "Multi Dut Cmd_Header Setting.vi"("WS1050/51"="WS1050/51", "Cmin/Act"="Cmin/Act", "Test Seq"="Test Sequences", "error in (no error)"=w752) -> ("Name 1"=w750:string[], "Name 2"=w749:string[], "Name Header"=w747:string[], "Name 3"=w748:string[], "Cmd 3"=w744:string[], "Cmd 1"=w746:string[], "Cmd 2"=w745:string[], "error out"=w753:errorcluster)  [unwired: 2 in, 2 out]
              }
              frame #1 {
                w1110 = FALSE ("Log (T)")
                n282 = call "WSVCAP SHL Host TL RFFE Configure.vi"("RFFE Slave Address"=w1121, "Clock Rate (Hz)"=w1119, "error in"=w1111) -> ("Actual Rate (Hz)"=w1129:dbl, "error out"=w1117:errorcluster)  [unwired: 11 in]
                n283 = local write "AR  Measurent(Hz)"(w1129) -> ()
                n284 = Array Size(array=w1122) -> (size(s)=w1132:i32)
                n285 = case shown="False" w1101 {
                  tunnel: w1132 -> [w1140 _]
                  tunnel: w1123 -> [w1139 _]
                  tunnel: w1122 -> [w1138 _]
                  tunnel: w1117 -> [w1137 w1226]
                  tunnel: [w1136 w1226] -> w1116
                  tunnel: w1110 -> [w1135 _]
                  tunnel: [w1134 string[][] []] -> w1105
                  tunnel: w1104 -> [w1133 _]
                  frame False {
                    n286 = case shown="2" w1133 {
                      tunnel: w1140 -> [w1147 w1175 w1203]
                      tunnel: w1139 -> [w1146 w1174 w1202]
                      tunnel: w1138 -> [w1145 w1173 w1201]
                      tunnel: w1137 -> [w1144 w1172 w1200]
                      tunnel: [w1143 w1171 w1199] -> w1136
                      tunnel: w1135 -> [w1142 w1170 w1198]
                      tunnel: [w1141 w1169 w1197] -> w1134
                      frame 0, Default {
                        n287 = for {
                          N: w1147 -> [_]
                          tunnel: w1146 -> [w1164]
                          tunnel: [w1160] -> w1141 mode=indexing
                          tunnel: w1145 -> [w1162]
                          tunnel: w1144 -> [w1150]
                          tunnel: [w1152] -> w1143
                          tunnel: w1142 -> [w1151]
                          i -> [w1159]
                          stop <- w1148 stop-if-true
                          n288 = Index Array(array=w1164, index=w1159) -> (element=w1163:string)
                          n289 = Index Array(array=w1162, index=w1159) -> (element=w1161:string)
                          n290 = local write "STATUS"(w1161) -> ()
                          n291 = call "WSVCAP SHL Host TL RFFE Write - Multiple DUTs - Common Data.vi"("Data Out"=w1163, "error in"=w1150, "Log (T)"=FALSE) -> ("error out"=w1154:errorcluster)  [unwired: 12 in]
                          n292 = call "Delay.vi"("milliseconds to wait"=u32 10, "error in (no error)"=w1154) -> ("error out"=w1158:errorcluster)  [unwired: 9 in]
                          n293 = call "WS1050 AD7747 READ 36 DUT.vi"("error in"=w1158, "Log (T)"=w1151, "DUT Mask Mode (All)"=WSVCAP_SHL_I2C_DUT_Mask_Mode_Enum."C1") -> ("error out"=w1156:errorcluster, "AD7747 Values"=w1157:string[][])  [unwired: 7 in]
                          n294 = for {
                            tunnel: w1157 -> [w1167] mode=indexing
                            tunnel: w1156 -> [w1168]
                            tunnel: [w1168] -> w1152
                            tunnel: [w1165] -> w1160 mode=indexing
                            n295 = Index Array(array=w1167, index=1) -> (element=w1165:string)
                          }
                          n296 = Unbundle By Name(w1152) -> ("status"=w1148:bool)
                        }
                      }
                      frame 1 {
                        n297 = for {
                          N: w1175 -> [_]
                          tunnel: w1174 -> [w1192]
                          tunnel: [w1188] -> w1169 mode=indexing
                          tunnel: w1173 -> [w1190]
                          tunnel: w1172 -> [w1178]
                          tunnel: [w1180] -> w1171
                          tunnel: w1170 -> [w1179]
                          i -> [w1187]
                          stop <- w1176 stop-if-true
                          n298 = Index Array(array=w1192, index=w1187) -> (element=w1191:string)
                          n299 = Index Array(array=w1190, index=w1187) -> (element=w1189:string)
                          n300 = local write "STATUS"(w1189) -> ()
                          n301 = call "WSVCAP SHL Host TL RFFE Write - Multiple DUTs - Common Data.vi"("Data Out"=w1191, "error in"=w1178, "Log (T)"=FALSE) -> ("error out"=w1182:errorcluster)  [unwired: 12 in]
                          n302 = call "Delay.vi"("milliseconds to wait"=u32 10, "error in (no error)"=w1182) -> ("error out"=w1186:errorcluster)  [unwired: 9 in]
                          n303 = call "WS1050 AD7747 READ 36 DUT.vi"("error in"=w1186, "Log (T)"=w1179, "DUT Mask Mode (All)"=WSVCAP_SHL_I2C_DUT_Mask_Mode_Enum."C2") -> ("error out"=w1184:errorcluster, "AD7747 Values"=w1185:string[][])  [unwired: 7 in]
                          n304 = for {
                            tunnel: w1185 -> [w1195] mode=indexing
                            tunnel: w1184 -> [w1196]
                            tunnel: [w1196] -> w1180
                            tunnel: [w1193] -> w1188 mode=indexing
                            n305 = Index Array(array=w1195, index=3) -> (element=w1193:string)
                          }
                          n306 = Unbundle By Name(w1180) -> ("status"=w1176:bool)
                        }
                      }
                      frame 2 {
                        n307 = for {
                          N: w1203 -> [_]
                          tunnel: w1202 -> [w1220]
                          tunnel: [w1216] -> w1197 mode=indexing
                          tunnel: w1201 -> [w1218]
                          tunnel: w1200 -> [w1206]
                          tunnel: [w1208] -> w1199
                          tunnel: w1198 -> [w1207]
                          i -> [w1215]
                          stop <- w1204 stop-if-true
                          n308 = Index Array(array=w1220, index=w1215) -> (element=w1219:string)
                          n309 = Index Array(array=w1218, index=w1215) -> (element=w1217:string)
                          n310 = local write "STATUS"(w1217) -> ()
                          n311 = call "WSVCAP SHL Host TL RFFE Write - Multiple DUTs - Common Data.vi"("Data Out"=w1219, "error in"=w1206, "Log (T)"=FALSE) -> ("error out"=w1210:errorcluster)  [unwired: 12 in]
                          n312 = call "Delay.vi"("milliseconds to wait"=u32 10, "error in (no error)"=w1210) -> ("error out"=w1214:errorcluster)  [unwired: 9 in]
                          n313 = call "WS1050 AD7747 READ 36 DUT.vi"("error in"=w1214, "Log (T)"=w1207, "DUT Mask Mode (All)"=WSVCAP_SHL_I2C_DUT_Mask_Mode_Enum."C3") -> ("error out"=w1212:errorcluster, "AD7747 Values"=w1213:string[][])  [unwired: 7 in]
                          n314 = for {
                            tunnel: w1213 -> [w1223] mode=indexing
                            tunnel: w1212 -> [w1224]
                            tunnel: [w1224] -> w1208
                            tunnel: [w1221] -> w1216 mode=indexing
                            n315 = Index Array(array=w1223, index=5) -> (element=w1221:string)
                          }
                          n316 = Unbundle By Name(w1208) -> ("status"=w1204:bool)
                        }
                      }
                    }
                  }
                  frame True {
                  }
                }
                n317 = Transpose 2D Array(2D array=w1105) -> (transposed array=w1115:string[][])
                "CAP_C1" <- w1115
                "NOM IDD ON (uA)" <- w1125
                "NOM IDD OFF(uA)" <- w1124
              }
              frame #2 {
                n318 = Array Size(array=w1244) -> (size(s)=w1245:i32)
                n319 = case shown="True" w1227 {
                  tunnel: w1245 -> [w1261 _]
                  tunnel: w1244 -> [w1260 _]
                  tunnel: w1243 -> [w1259 _]
                  tunnel: [w1258 w1319] -> w1241
                  tunnel: w1239 -> [w1257 w1319]
                  tunnel: w1233 -> [w1256 _]
                  tunnel: [w1255 string[][] []] -> w1231
                  tunnel: w1230 -> [w1254 _]
                  frame False {
                    n320 = case shown="0, 2, Default" w1254 {
                      tunnel: w1261 -> [w1268 w1296]
                      tunnel: w1260 -> [w1267 w1295]
                      tunnel: w1259 -> [w1266 w1294]
                      tunnel: [w1265 w1293] -> w1258
                      tunnel: w1257 -> [w1264 w1292]
                      tunnel: w1256 -> [w1263 w1291]
                      tunnel: [w1262 w1290] -> w1255
                      frame 0, 2, Default {
                        n321 = for {
                          N: w1268 -> [_]
                          tunnel: w1266 -> [w1285]
                          tunnel: [w1281] -> w1262 mode=indexing
                          tunnel: w1267 -> [w1283]
                          tunnel: w1264 -> [w1271]
                          tunnel: [w1273] -> w1265
                          tunnel: w1263 -> [w1272]
                          i -> [w1280]
                          stop <- w1269 stop-if-true
                          n322 = Index Array(array=w1285, index=w1280) -> (element=w1284:string)
                          n323 = Index Array(array=w1283, index=w1280) -> (element=w1282:string)
                          n324 = call "WSVCAP SHL Host TL RFFE Write - Multiple DUTs - Common Data.vi"("Data Out"=w1284, "error in"=w1271, "Log (T)"=FALSE) -> ("error out"=w1275:errorcluster)  [unwired: 12 in]
                          n325 = local write "STATUS"(w1282) -> ()
                          n326 = call "Delay.vi"("milliseconds to wait"=u32 10, "error in (no error)"=w1275) -> ("error out"=w1279:errorcluster)  [unwired: 9 in]
                          n327 = call "WS1050 AD7747 READ 36 DUT.vi"("error in"=w1279, "Log (T)"=w1272, "DUT Mask Mode (All)"=WSVCAP_SHL_I2C_DUT_Mask_Mode_Enum."C2") -> ("error out"=w1277:errorcluster, "AD7747 Values"=w1278:string[][])  [unwired: 7 in]
                          n328 = for {
                            tunnel: w1278 -> [w1288] mode=indexing
                            tunnel: w1277 -> [w1289]
                            tunnel: [w1289] -> w1273
                            tunnel: [w1286] -> w1281 mode=indexing
                            n329 = Index Array(array=w1288, index=3) -> (element=w1286:string)
                          }
                          n330 = Unbundle By Name(w1273) -> ("status"=w1269:bool)
                        }
                      }
                      frame 1 {
                        n331 = for {
                          N: w1296 -> [_]
                          tunnel: w1294 -> [w1313]
                          tunnel: [w1309] -> w1290 mode=indexing
                          tunnel: w1295 -> [w1311]
                          tunnel: w1292 -> [w1299]
                          tunnel: [w1301] -> w1293
                          tunnel: w1291 -> [w1300]
                          i -> [w1308]
                          stop <- w1297 stop-if-true
                          n332 = Index Array(array=w1313, index=w1308) -> (element=w1312:string)
                          n333 = Index Array(array=w1311, index=w1308) -> (element=w1310:string)
                          n334 = call "WSVCAP SHL Host TL RFFE Write - Multiple DUTs - Common Data.vi"("Data Out"=w1312, "error in"=w1299, "Log (T)"=FALSE) -> ("error out"=w1303:errorcluster)  [unwired: 12 in]
                          n335 = local write "STATUS"(w1310) -> ()
                          n336 = call "Delay.vi"("milliseconds to wait"=u32 10, "error in (no error)"=w1303) -> ("error out"=w1307:errorcluster)  [unwired: 9 in]
                          n337 = call "WS1050 AD7747 READ 36 DUT.vi"("error in"=w1307, "Log (T)"=w1300, "DUT Mask Mode (All)"=WSVCAP_SHL_I2C_DUT_Mask_Mode_Enum."C1") -> ("error out"=w1305:errorcluster, "AD7747 Values"=w1306:string[][])  [unwired: 7 in]
                          n338 = for {
                            tunnel: w1306 -> [w1316] mode=indexing
                            tunnel: w1305 -> [w1317]
                            tunnel: [w1317] -> w1301
                            tunnel: [w1314] -> w1309 mode=indexing
                            n339 = Index Array(array=w1316, index=1) -> (element=w1314:string)
                          }
                          n340 = Unbundle By Name(w1301) -> ("status"=w1297:bool)
                        }
                      }
                    }
                  }
                  frame True {
                  }
                }
                n341 = Transpose 2D Array(2D array=w1231) -> (transposed array=w1240:string[][])
                "CAP_C2" <- w1240
              }
              frame #3 {
                n342 = Array Size(array=w1337) -> (size(s)=w1338:i32)
                n343 = case shown="True" w1320 {
                  tunnel: w1338 -> [w1355 _]
                  tunnel: w1337 -> [w1354 _]
                  tunnel: w1336 -> [w1353 _]
                  tunnel: w1331 -> [w1352 w1413]
                  tunnel: w1327 -> [w1351 _]
                  tunnel: [w1350 string[][] []] -> w1325
                  tunnel: w1324 -> [w1349 _]
                  tunnel: [w1348 w1413] -> w1323
                  frame False {
                    n344 = case shown="2" w1349 {
                      tunnel: w1355 -> [w1362 w1390]
                      tunnel: w1354 -> [w1361 w1389]
                      tunnel: w1353 -> [w1360 w1388]
                      tunnel: w1352 -> [w1359 w1387]
                      tunnel: [w1358 w1386] -> w1348
                      tunnel: w1351 -> [w1357 w1385]
                      tunnel: [w1356 w1384] -> w1350
                      frame 0, 1, Default {
                        n345 = for {
                          N: w1362 -> [_]
                          tunnel: w1360 -> [w1379]
                          tunnel: [w1375] -> w1356 mode=indexing
                          tunnel: w1361 -> [w1377]
                          tunnel: w1359 -> [w1365]
                          tunnel: [w1367] -> w1358
                          tunnel: w1357 -> [w1366]
                          i -> [w1374]
                          stop <- w1363 stop-if-true
                          n346 = Index Array(array=w1379, index=w1374) -> (element=w1378:string)
                          n347 = Index Array(array=w1377, index=w1374) -> (element=w1376:string)
                          n348 = local write "STATUS"(w1376) -> ()
                          n349 = call "WSVCAP SHL Host TL RFFE Write - Multiple DUTs - Common Data.vi"("Data Out"=w1378, "error in"=w1365, "Log (T)"=FALSE) -> ("error out"=w1369:errorcluster)  [unwired: 12 in]
                          n350 = call "Delay.vi"("milliseconds to wait"=u32 10, "error in (no error)"=w1369) -> ("error out"=w1373:errorcluster)  [unwired: 9 in]
                          n351 = call "WS1050 AD7747 READ 36 DUT.vi"("error in"=w1373, "Log (T)"=w1366, "DUT Mask Mode (All)"=WSVCAP_SHL_I2C_DUT_Mask_Mode_Enum."C3") -> ("error out"=w1371:errorcluster, "AD7747 Values"=w1372:string[][])  [unwired: 7 in]
                          n352 = for {
                            tunnel: w1372 -> [w1382] mode=indexing
                            tunnel: w1371 -> [w1383]
                            tunnel: [w1383] -> w1367
                            tunnel: [w1380] -> w1375 mode=indexing
                            n353 = Index Array(array=w1382, index=5) -> (element=w1380:string)
                          }
                          n354 = Unbundle By Name(w1367) -> ("status"=w1363:bool)
                        }
                      }
                      frame 2 {
                        n355 = for {
                          N: w1390 -> [_]
                          tunnel: w1388 -> [w1407]
                          tunnel: [w1403] -> w1384 mode=indexing
                          tunnel: w1389 -> [w1405]
                          tunnel: w1387 -> [w1393]
                          tunnel: [w1395] -> w1386
                          tunnel: w1385 -> [w1394]
                          i -> [w1402]
                          stop <- w1391 stop-if-true
                          n356 = Index Array(array=w1407, index=w1402) -> (element=w1406:string)
                          n357 = Index Array(array=w1405, index=w1402) -> (element=w1404:string)
                          n358 = local write "STATUS"(w1404) -> ()
                          n359 = call "WSVCAP SHL Host TL RFFE Write - Multiple DUTs - Common Data.vi"("Data Out"=w1406, "error in"=w1393, "Log (T)"=FALSE) -> ("error out"=w1397:errorcluster)  [unwired: 12 in]
                          n360 = call "Delay.vi"("milliseconds to wait"=u32 10, "error in (no error)"=w1397) -> ("error out"=w1401:errorcluster)  [unwired: 9 in]
                          n361 = call "WS1050 AD7747 READ 36 DUT.vi"("error in"=w1401, "Log (T)"=w1394, "DUT Mask Mode (All)"=WSVCAP_SHL_I2C_DUT_Mask_Mode_Enum."C1") -> ("error out"=w1399:errorcluster, "AD7747 Values"=w1400:string[][])  [unwired: 7 in]
                          n362 = for {
                            tunnel: w1400 -> [w1410] mode=indexing
                            tunnel: w1399 -> [w1411]
                            tunnel: [w1411] -> w1395
                            tunnel: [w1408] -> w1403 mode=indexing
                            n363 = Index Array(array=w1410, index=1) -> (element=w1408:string)
                          }
                          n364 = Unbundle By Name(w1395) -> ("status"=w1391:bool)
                        }
                      }
                    }
                  }
                  frame True {
                  }
                }
                n365 = Transpose 2D Array(2D array=w1325) -> (transposed array=w1332:string[][])
                "CAP_C3" <- w1332
              }
              frame #4 {
                # "VPI Testing @ 35V"
                n366 = call "WS1050 Delta C Calculation.vi"("error in (no error)"=w1455, "DCap Target(pF)"=w1454, "Input"=w1457) -> ("error out"=w1452:errorcluster, "Total Bank Delta C(pF)"=w1445:string[], "% Bank DeltaC"=w1449:string[])  [unwired: 4 in, 2 out]
                n367 = call "WS1050 Delta C Calculation.vi"("error in (no error)"=w1455, "DCap Target(pF)"=w1454, "Input"=w1456) -> ("error out"=w1453:errorcluster, "Total Bank Delta C(pF)"=w1444:string[], "% Bank DeltaC"=w1447:string[])  [unwired: 4 in, 2 out]
                n368 = call "WS1050 Delta C Calculation.vi"("error in (no error)"=w1455, "DCap Target(pF)"=w1454, "Input"=w1448) -> ("error out"=w1451:errorcluster, "Total Bank Delta C(pF)"=w1443:string[], "% Bank DeltaC"=w1446:string[])  [unwired: 4 in, 2 out]
                n369 = Merge Errors(w1452, w1453, w1451) -> (w1450:errorcluster)
                n370 = case shown="1, Default" w1458 {
                  tunnel: w1450 -> [w1656 w1664]
                  tunnel: [w1656 w1664] -> w1417
                  tunnel: w1449 -> [w1652 w1660]
                  tunnel: w1447 -> [w1651 w1659]
                  tunnel: w1446 -> [w1650 w1658]
                  tunnel: w1445 -> [w1655 w1663]
                  tunnel: [w1655 w1663] -> w1442
                  tunnel: w1444 -> [w1654 w1662]
                  tunnel: [w1654 w1662] -> w1441
                  tunnel: w1443 -> [w1653 w1661]
                  tunnel: [w1653 w1661] -> w1440
                  frame 0 {
                    n371 = Build Array(w1652, w1651, w1650) -> (→"% Delta C_T0":string[][])
                  }
                  frame 1, Default {
                    n372 = Build Array(w1660, w1659, w1658) -> (→"% Delta C":string[][])
                  }
                }
                "Total Delta C1(pF)" <- w1442
                "Total Delta C2(pF)" <- w1441
                "Total Delta C3(pF)" <- w1440
                n373 = call "WS1050_51 VPI Header.vi"("VPI Name"="VPI Name", "VPI_Cmd"="VPI_Cmd", "Cmin/Act"=w1415, "WS1050/51"=w1426, "error in (no error)"=w1427) -> ("VPI_1"=w1425:string[], "VPI_2"=w1423:string[], "VPI Header"=w1424:string[], "VPI_3"=w1422:string[], "Cmd_3"=w1419:string[], "Cmd_1"=w1421:string[], "Cmd_2"=w1420:string[], "error out"=w1418:errorcluster)  [unwired: 3 in]
                n374 = Merge Errors(w1418, w1417) -> (w1416:errorcluster)
                n375 = case shown="False" w1414 {
                  tunnel: [w1485 w1640] -> w1470
                  tunnel: [w1484 w1640] -> w1469
                  tunnel: w1465 -> [w1483 w1638]
                  tunnel: [w1482 w1638] -> w1464
                  tunnel: [w1481 w1640] -> w1461
                  tunnel: [w1480 "" ("Data Out")] -> w1438
                  tunnel: [w1479 w1639] -> w1436
                  tunnel: w1432 -> [w1478 _]
                  tunnel: w1425 -> [w1477 _]
                  tunnel: w1423 -> [w1476 _]
                  tunnel: w1422 -> [w1475 _]
                  tunnel: w1421 -> [w1474 _]
                  tunnel: w1420 -> [w1473 _]
                  tunnel: w1419 -> [w1472 _]
                  tunnel: w1416 -> [w1471 w1639]
                  frame False {
                    n376 = case shown="False" w1478 {
                      tunnel: [w1488 w1509] -> w1479
                      tunnel: [w1486 w1527] -> w1485
                      tunnel: [w1486 w1513] -> w1484
                      tunnel: w1483 -> [w1493 w1526]
                      tunnel: [w1493 w1526] -> w1482
                      tunnel: w1474 -> [_ w1525]
                      tunnel: w1473 -> [_ w1519]
                      tunnel: w1472 -> [_ w1515]
                      tunnel: [w1486 w1524] -> w1481
                      tunnel: w1477 -> [w1491 w1522]
                      tunnel: w1476 -> [_ w1520]
                      tunnel: w1475 -> [_ w1516]
                      tunnel: ["NA" ("string") w1503] -> w1480
                      tunnel: w1471 -> [w1489 w1507]
                      frame False {
                        n377 = Array Size(array=w1491) -> (size(s)=w1490:i32)
                        n378 = for {
                          N: w1490 -> [_]
                          tunnel: [w1495] -> w1487 mode=indexing
                          tunnel: w1489 -> [w1494]
                          tunnel: [w1494] -> w1488
                          n379 = for {
                            N: 36 -> [_]
                            tunnel: [""] -> w1495 mode=indexing
                          }
                        }
                        n380 = Transpose 2D Array(2D array=w1487) -> (transposed array=w1486:string[][])
                        n381 = local write "VPI C1"(w1486) -> ()
                        n382 = local write "VPI C2"(w1486) -> ()
                        n383 = local write "VPI C3"(w1486) -> ()
                      }
                      frame True {
                        w1508 = FALSE ("Log (T)")
                        # "Set CP VPI"
                        n384 = call "WSVCAP SHL Host TL RFFE Write - Multiple DUTs - Common Data.vi"("Data Out"="074820", "error in"=w1507, "Log (T)"=w1508) -> ("error out"=w1505:errorcluster)  [unwired: 12 in]
                        n385 = call "Delay.vi"("milliseconds to wait"=u32 10, "error in (no error)"=w1505) -> ("error out"=w1501:errorcluster)  [unwired: 9 in]
                        n386 = case shown="0, Default" "CP VPI" {
                          selector: "CP VPI" -> [w1532 w1537 w1542 w1547 w1552 w1557 w1562 w1567 w1571]
                          tunnel: string[] ["07476F", "074776", "074765", "074769", "07477B", "07477C", "07477D", "074779", "07476B"] -> [w1533 w1538 w1543 w1548 w1553 w1558 w1563 w1568 w1573]
                          tunnel: [w1531 w1536 w1541 w1546 w1551 w1556 w1561 w1566 w1572] -> w1500
                          tunnel: ["35.0" ("Data Out") "27.5" ("Data Out") "30.5" ("Data Out") "44.0" ("Data Out") "50.0" ("Data Out") "55.0" ("Data Out") "42.5" ("Data Out") "32.0" ("Data Out") "40.25" ("Data Out")] -> w1503
                          tunnel: [w1529 w1534 w1539 w1544 w1549 w1554 w1559 w1564 w1569] -> w1502
                          tunnel: w1501 -> [w1529 w1534 w1539 w1544 w1549 w1554 w1559 w1564 w1569]
                          frame 0, Default {
                            n387 = Index Array(array=w1533, index=w1532) -> (element=w1531:string)
                          }
                          frame 2 {
                            n388 = Index Array(array=w1538, index=w1537) -> (element=w1536:string)
                          }
                          frame 3 {
                            n389 = Index Array(array=w1543, index=w1542) -> (element=w1541:string)
                          }
                          frame 4 {
                            n390 = Index Array(array=w1548, index=w1547) -> (element=w1546:string)
                          }
                          frame 5 {
                            n391 = Index Array(array=w1553, index=w1552) -> (element=w1551:string)
                          }
                          frame 6 {
                            n392 = Index Array(array=w1558, index=w1557) -> (element=w1556:string)
                          }
                          frame 7 {
                            n393 = Index Array(array=w1563, index=w1562) -> (element=w1561:string)
                          }
                          frame 8 {
                            n394 = Index Array(array=w1568, index=w1567) -> (element=w1566:string)
                          }
                          frame 1 {
                            n395 = Index Array(array=w1573, index=w1571) -> (element=w1572:string)
                          }
                        }
                        n396 = Array Size(array=w1522) -> (size(s)=w1528:i32)
                        n397 = call "WSVCAP SHL Host TL RFFE Write - Multiple DUTs - Common Data.vi"("Data Out"=w1500, "error in"=w1502, "Log (T)"=w1508) -> ("error out"=w1512:errorcluster)  [unwired: 12 in]
                        n398 = for {
                          N: w1528 -> [_]
                          tunnel: w1525 -> [w1632]
                          tunnel: [w1630] -> w1523 mode=indexing
                          tunnel: w1522 -> [w1629]
                          tunnel: w1512 -> [w1618]
                          tunnel: [w1620] -> w1511
                          i -> [w1628]
                          stop <- w1616 stop-if-true
                          n399 = Index Array(array=w1632, index=w1628) -> (element=w1631:string)
                          n400 = Index Array(array=w1629, index=w1628) -> (element=w1627:string)
                          n401 = local write "STATUS"(w1627) -> ()
                          n402 = call "WSVCAP SHL Host TL RFFE Write - Multiple DUTs - Common Data.vi"("Data Out"=w1631, "error in"=w1618, "Log (T)"=FALSE) -> ("error out"=w1626:errorcluster)  [unwired: 12 in]
                          n403 = call "Delay.vi"("milliseconds to wait"=u32 10, "error in (no error)"=w1626) -> ("error out"=w1622:errorcluster)  [unwired: 9 in]
                          n404 = call "WS1050 AD7747 READ 36 DUT.vi"("error in"=w1622, "Log (T)"=FALSE, "DUT Mask Mode (All)"=WSVCAP_SHL_I2C_DUT_Mask_Mode_Enum."C1") -> ("error out"=w1624:errorcluster, "AD7747 Values"=w1623:string[][])  [unwired: 7 in]
                          n405 = for {
                            tunnel: [w1635] -> w1630 mode=indexing
                            tunnel: w1624 -> [w1634]
                            tunnel: [w1634] -> w1620
                            tunnel: w1623 -> [w1633] mode=indexing
                            n406 = Index Array(array=w1633, index=1) -> (element=w1635:string)
                          }
                          n407 = Unbundle By Name(w1620) -> ("status"=w1616:bool)
                        }
                        n408 = Transpose 2D Array(2D array=w1523) -> (transposed array=w1527:string[][])
                        "VPI C1" <- w1527
                        n409 = Array Size(array=w1520) -> (size(s)=w1521:i32)
                        n410 = for {
                          N: w1521 -> [_]
                          tunnel: w1519 -> [w1611]
                          tunnel: [w1609] -> w1518 mode=indexing
                          tunnel: w1520 -> [w1608]
                          tunnel: w1511 -> [w1597]
                          tunnel: [w1599] -> w1510
                          i -> [w1607]
                          stop <- w1595 stop-if-true
                          n411 = Index Array(array=w1611, index=w1607) -> (element=w1610:string)
                          n412 = Index Array(array=w1608, index=w1607) -> (element=w1606:string)
                          n413 = call "WSVCAP SHL Host TL RFFE Write - Multiple DUTs - Common Data.vi"("Data Out"=w1610, "error in"=w1597, "Log (T)"=FALSE) -> ("error out"=w1605:errorcluster)  [unwired: 12 in]
                          n414 = local write "STATUS"(w1606) -> ()
                          n415 = call "Delay.vi"("milliseconds to wait"=u32 10, "error in (no error)"=w1605) -> ("error out"=w1601:errorcluster)  [unwired: 9 in]
                          n416 = call "WS1050 AD7747 READ 36 DUT.vi"("error in"=w1601, "Log (T)"=FALSE, "DUT Mask Mode (All)"=WSVCAP_SHL_I2C_DUT_Mask_Mode_Enum."C2") -> ("error out"=w1603:errorcluster, "AD7747 Values"=w1602:string[][])  [unwired: 7 in]
                          n417 = for {
                            tunnel: [w1614] -> w1609 mode=indexing
                            tunnel: w1603 -> [w1613]
                            tunnel: [w1613] -> w1599
                            tunnel: w1602 -> [w1612] mode=indexing
                            n418 = Index Array(array=w1612, index=3) -> (element=w1614:string)
                          }
                          n419 = Unbundle By Name(w1599) -> ("status"=w1595:bool)
                        }
                        n420 = Transpose 2D Array(2D array=w1518) -> (transposed array=w1524:string[][])
                        "VPI C2" <- w1524
                        n421 = Array Size(array=w1516) -> (size(s)=w1517:i32)
                        n422 = for {
                          N: w1517 -> [_]
                          tunnel: w1515 -> [w1590]
                          tunnel: [w1588] -> w1514 mode=indexing
                          tunnel: w1516 -> [w1587]
                          tunnel: w1510 -> [w1576]
                          tunnel: [w1578] -> w1509
                          i -> [w1586]
                          stop <- w1574 stop-if-true
                          n423 = Index Array(array=w1590, index=w1586) -> (element=w1589:string)
                          n424 = Index Array(array=w1587, index=w1586) -> (element=w1585:string)
                          n425 = call "WSVCAP SHL Host TL RFFE Write - Multiple DUTs - Common Data.vi"("Data Out"=w1589, "error in"=w1576, "Log (T)"=FALSE) -> ("error out"=w1584:errorcluster)  [unwired: 12 in]
                          n426 = local write "STATUS"(w1585) -> ()
                          n427 = call "Delay.vi"("milliseconds to wait"=u32 10, "error in (no error)"=w1584) -> ("error out"=w1580:errorcluster)  [unwired: 9 in]
                          n428 = call "WS1050 AD7747 READ 36 DUT.vi"("error in"=w1580, "Log (T)"=FALSE, "DUT Mask Mode (All)"=WSVCAP_SHL_I2C_DUT_Mask_Mode_Enum."C3") -> ("error out"=w1582:errorcluster, "AD7747 Values"=w1581:string[][])  [unwired: 7 in]
                          n429 = for {
                            tunnel: [w1593] -> w1588 mode=indexing
                            tunnel: w1582 -> [w1592]
                            tunnel: [w1592] -> w1578
                            tunnel: w1581 -> [w1591] mode=indexing
                            n430 = Index Array(array=w1591, index=5) -> (element=w1593:string)
                          }
                          n431 = Unbundle By Name(w1578) -> ("status"=w1574:bool)
                        }
                        n432 = Transpose 2D Array(2D array=w1514) -> (transposed array=w1513:string[][])
                        "VPI C3" <- w1513
                      }
                    }
                  }
                  frame True {
                    w1640 = string[][] []
                  }
                }
                n433 = Insert Into Array(array=w1460, new element=w1424) -> (w1459:string[])  [unwired: 1 in]
                n434 = case shown="True" w1437 {
                  tunnel: w1436 -> [w1642 w1647]
                  tunnel: [w1643 w1646] -> w1435
                  frame False {
                    n435 = call "WSVCAP SHL Host TL RFFE Write - Multiple DUTs - Common Data.vi"("Data Out"="074820", "error in"=w1642, "Log (T)"=FALSE) -> ("error out"=w1643:errorcluster)  [unwired: 12 in]
                  }
                  frame True {
                    n436 = call "WSVCAP SHL Host TL RFFE Write - Multiple DUTs - Common Data.vi"("Data Out"="074800", "error in"=w1647, "Log (T)"=FALSE) -> ("error out"=w1646:errorcluster)  [unwired: 12 in]
                  }
                }
                n437 = call "Delay.vi"("milliseconds to wait"=u32 10, "error in (no error)"=w1435) -> ("error out"=w1434:errorcluster)  [unwired: 9 in]
              }
              frame #5 {
                # "VSA Testing"
                n438 = case shown="True" w1665 {
                  tunnel: w1705 -> [w1715 w1785]
                  tunnel: w1696 -> [w1714 w1784]
                  tunnel: [w1713 w1784] -> w1695
                  tunnel: [w1712 string[][] []] -> w1685
                  tunnel: [w1711 w1786] -> w1684
                  tunnel: [w1710 w1786] -> w1681
                  tunnel: [w1709 w1785] -> w1679
                  tunnel: [w1708 w1786] -> w1678
                  tunnel: w1666 -> [w1707 _]
                  frame False {
                    n439 = case shown="True" w1707 {
                      tunnel: w1715 -> [w1717 w1731]
                      tunnel: [w1716 w1730] -> w1709
                      tunnel: [w1721 w1737] -> w1713
                      tunnel: w1714 -> [w1721 w1736]
                      tunnel: [w1718 w1734] -> w1711
                      tunnel: [w1718 w1733] -> w1710
                      tunnel: [w1718 w1732] -> w1708
                      tunnel: [w1719 w1735] -> w1712
                      frame False {
                        n440 = for {
                          tunnel: dbl[] [0.0, 0.0, 0.0] -> [w1726] mode=indexing
                          tunnel: [w1725] -> w1719 mode=indexing
                          tunnel: [w1722] -> w1718 mode=indexing
                          tunnel: w1717 -> [w1723]
                          tunnel: [w1723] -> w1716
                          n441 = Number To Fractional String(number=w1726) -> (F-format string=w1727:string)  [unwired: 3 in]
                          n442 = for {
                            N: 36 -> [_]
                            tunnel: w1727 -> [w1729]
                            tunnel: [w1729] -> w1725 mode=indexing
                            tunnel: [""] -> w1722 mode=indexing
                          }
                        }
                      }
                      frame True {
                        n443 = for {
                          tunnel: "VSA Voltage(V)" -> [w1761] mode=indexing
                          tunnel: [w1765] -> w1737
                          tunnel: w1736 -> [w1763]
                          tunnel: [w1762] -> w1734 mode=indexing
                          tunnel: [w1749] -> w1733 mode=indexing
                          tunnel: [w1758] -> w1735 mode=indexing
                          tunnel: [w1743] -> w1732 mode=indexing
                          tunnel: w1731 -> [w1742]
                          tunnel: [w1741] -> w1730
                          w1740 = FALSE ("Log (T)")
                          w1757 = u16 0 items=["Voltage", "Current"] ("Source Mode  (0: Voltage)")
                          n444 = call "Ke2400 Configure Output.vi"("Source Mode  (0: Voltage)"=w1757, "error in (no error)"=w1742, "Compliance  Level (0.1)"=0.1, "Output Level (0)"=w1761, "VISA resource name"=w1763) -> ("error out"=w1769:errorcluster, "VISA resource name out"=w1767:refnum<visa-resource-name>)  [unwired: 5 in]
                          n445 = Number To Fractional String(number=w1761) -> (F-format string=w1760:string)  [unwired: 3 in]
                          n446 = call "Ke2400 Enable.vi"("error in (no error)"=w1769, "ON/OFF"=TRUE ("Enable Output (T: Enable)"), "VISA resource name"=w1767) -> ("error out"=w1770:errorcluster, "VISA resource name out"=w1765:refnum<visa-resource-name>)  [unwired: 7 in]
                          n447 = call "Delay.vi"("milliseconds to wait"=u32 10, "error in (no error)"=w1770) -> ("error out"=w1756:errorcluster)  [unwired: 9 in]
                          n448 = call "WS1050 AD7747 READ 36 DUT.vi"("error in"=w1756, "Log (T)"=w1740, "DUT Mask Mode (All)"=WSVCAP_SHL_I2C_DUT_Mask_Mode_Enum."C1") -> ("error out"=w1753:errorcluster, "AD7747 Values"=w1755:string[][])  [unwired: 7 in]
                          n449 = for {
                            tunnel: w1755 -> [w1781] mode=indexing
                            tunnel: [w1782] -> w1762 mode=indexing
                            tunnel: w1753 -> [w1780]
                            tunnel: [w1780] -> w1752
                            n450 = Index Array(array=w1781, index=1) -> (element=w1782:string)
                          }
                          n451 = for {
                            N: 36 -> [_]
                            tunnel: w1760 -> [w1779]
                            tunnel: [w1779] -> w1758 mode=indexing
                          }
                          n452 = call "WS1050 AD7747 READ 36 DUT.vi"("error in"=w1752, "Log (T)"=w1740, "DUT Mask Mode (All)"=WSVCAP_SHL_I2C_DUT_Mask_Mode_Enum."C2") -> ("error out"=w1750:errorcluster, "AD7747 Values"=w1748:string[][])  [unwired: 7 in]
                          n453 = for {
                            tunnel: w1748 -> [w1776] mode=indexing
                            tunnel: [w1777] -> w1749 mode=indexing
                            tunnel: w1750 -> [w1775]
                            tunnel: [w1775] -> w1747
                            n454 = Index Array(array=w1776, index=3) -> (element=w1777:string)
                          }
                          n455 = call "WS1050 AD7747 READ 36 DUT.vi"("error in"=w1747, "Log (T)"=w1740, "DUT Mask Mode (All)"=WSVCAP_SHL_I2C_DUT_Mask_Mode_Enum."C3") -> ("error out"=w1745:errorcluster, "AD7747 Values"=w1744:string[][])  [unwired: 7 in]
                          n456 = local write "STATUS"("VSA Testing...." ("STATUS")) -> ()
                          n457 = for {
                            tunnel: w1744 -> [w1772] mode=indexing
                            tunnel: [w1773] -> w1743 mode=indexing
                            tunnel: w1745 -> [w1771]
                            tunnel: [w1771] -> w1741
                            n458 = Index Array(array=w1772, index=5) -> (element=w1773:string)
                          }
                        }
                      }
                    }
                  }
                  frame True {
                    w1786 = string[][] []
                  }
                }
                n459 = Transpose 2D Array(2D array=w1685) -> (transposed array=w1683:string[][])
                n460 = Transpose 2D Array(2D array=w1684) -> (transposed array=w1682:string[][])
                n461 = Transpose 2D Array(2D array=w1681) -> (transposed array=w1680:string[][])
                n462 = Transpose 2D Array(2D array=w1678) -> (transposed array=w1677:string[][])
                n463 = call "WS1050_VSA_Convert_Data.vi"("VSA_C3"=w1677, "error in (no error)"=w1679, "VSA_C2"=w1680, "VSA_C1"=w1682, "Voltage"=w1683) -> ("error out"=w1676:errorcluster, "VSA_V3"=w1673:string[][], "VSA_V2"=w1674:string[][], "VSA_V1"=w1675:string[][])  [unwired: 3 in]
                "VSA_V1" <- w1675
                "VSA_V2" <- w1674
                "VSA_V3" <- w1673
                n464 = case shown="True" w1666 {
                  tunnel: w1695 -> [w1789 w1795]
                  tunnel: [w1789 w1794] -> w1694
                  tunnel: w1676 -> [w1788 w1793]
                  tunnel: [w1788 w1790] -> w1693
                  frame False {
                  }
                  frame True {
                    w1791 = u16 0 items=["Voltage", "Current"] ("Source Mode  (0: Voltage)")
                    n465 = call "Ke2400 Configure Output.vi"("Source Mode  (0: Voltage)"=w1791, "error in (no error)"=w1793, "Output Level (0)"=0.0, "VISA resource name"=w1795) -> ("error out"=w1790:errorcluster, "VISA resource name out"=w1794:refnum<visa-resource-name>)  [unwired: 6 in]
                  }
                }
                n466 = call "Delay.vi"("milliseconds to wait"=u32 50, "error in (no error)"=w1693) -> ("error out"=w1692:errorcluster)  [unwired: 9 in]
              }
              frame #6 {
                # "Handshake Check and EFuse Readback"
                n467 = Or(x=w1804, y=w1814) -> (x .or. y?=w1813:bool)
                n468 = Add(x=w1826, y=w1825) -> (x+y=w1812:u64)
                n469 = case shown="True" w1813 {
                  tunnel: w1839 -> [w1852 _]
                  tunnel: w1838 -> [w1851 w1857]
                  tunnel: [w1850 w1857] -> w1837
                  tunnel: w1836 -> [w1849 _]
                  tunnel: w1835 -> [w1848 _]
                  tunnel: w1834 -> [w1847 _]
                  tunnel: [w1843 w1856] -> w1833
                  tunnel: [w1842 w1856] -> w1828
                  tunnel: w1812 -> [w1841 _]
                  tunnel: w1819 -> [w1840 _]
                  frame False {
                    n470 = call "WS1050_36DUT_Handshake Check R1_Record All Regs Ver1.0.vi"("file path (use dialog)"=w1852, "Reg1_Bit Cntrl"="Reg1_Bit Cntrl", "File Name"=w1840, "SN"=w1847, "Loop"=w1841, "error"=w1851, "Lot #"=w1849, "Wafer #"=w1848) -> ("Pass/Fail"=→"EFuse Readback Status":bool[], "EFuse Read back"=w1842:string[], "Status"=w1843:string[], "error out"=w1850:errorcluster)  [unwired: 6 in, 2 out]
                    n471 = case shown="1, Default" w1841 {
                      tunnel: w1842 -> [w1853 w1854]
                      frame 0 {
                        "EFuse RB T0" <- w1853
                      }
                      frame 1, Default {
                        "Current EFuse Read back" <- w1854
                      }
                    }
                    n472 = local write "STATUS"("Hand Shake & EFuse Readback...." ("STATUS")) -> ()
                  }
                  frame True {
                    n473 = for {
                      N: 36 -> [_]
                      tunnel: [""] -> w1856 mode=indexing
                    }
                  }
                }
                n474 = Add(x=w1812, y=w1809) -> (x+y=w1810:u64)
                "TTCompleted" <- w1810
                n475 = Number To Engineering String(4:w1810) -> (0:w1824:string)  [unwired: 3 in]
                n476 = Build Array(w1823, w1821, w1820) -> (w1822:string[])
              }
              frame #7 {
                # "Save Data"
                n477 = Increment(x=w1871) -> (x+1=w1870:i32)
                n478 = Multiply(x=w1870, y=36) -> (x*y=w1865:i32)
                n479 = Path To String(path=w1875) -> (string=w1874:string)
                n480 = Bundle("Test Program"=w1906, "Comment"=w1905, "Data Out"=w1882, "Data Out"=w1881, "Data Out"=w1880, w1879, "Data Out"=w1878, "Data Out"=w1877, "Data Out"=w1876, "Freq(Hz)"=w1863, "Board#"=w1861) -> (w1862:T8)  [unwired: 1 in]
                n481 = case shown="True" w1860 {
                  tunnel: w1911 -> [w1938 w1940]
                  tunnel: [w1937 w1940] -> w1910
                  tunnel: w1909 -> [w1936 _]
                  tunnel: w1908 -> [w1935 _]
                  tunnel: w1907 -> [w1934 _]
                  tunnel: w1904 -> [w1933 _]
                  tunnel: w1902 -> [w1932 _]
                  tunnel: w1901 -> [w1931 _]
                  tunnel: w1900 -> [w1930 _]
                  tunnel: w1899 -> [w1929 _]
                  tunnel: w1898 -> [w1928 _]
                  tunnel: w1895 -> [w1927 _]
                  tunnel: w1894 -> [w1926 _]
                  tunnel: w1893 -> [w1925 _]
                  tunnel: w1891 -> [w1924 _]
                  tunnel: w1890 -> [w1923 _]
                  tunnel: w1889 -> [w1922 _]
                  tunnel: w1888 -> [w1921 _]
                  tunnel: w1887 -> [w1920 _]
                  tunnel: w1886 -> [w1919 _]
                  tunnel: w1885 -> [w1918 _]
                  tunnel: w1884 -> [w1917 _]
                  tunnel: w1883 -> [w1916 _]
                  tunnel: w1875 -> [w1915 _]
                  tunnel: w1868 -> [w1914 _]
                  tunnel: w1862 -> [w1913 _]
                  tunnel: ["Save Data...." ("STATUS") "Stop test..." ("STATUS")] -> w1859
                  frame False {
                    n482 = call "WS1050_36 DUT SData Ver1.0.vi"("TMN DC\\CAP Data Log File Path"=w1915, "Lot#"=w1935, "Total Delta C1(pF)"=w1918, "VSA_V1"=w1926, "Wafer#"=w1933, "File Name"=w1914, "Total Delta C2(pF)"=w1917, "error in"=w1938, "TP/Comment"=w1913, "EFuse"=w1929, "Data Output C3"=w1920, "Temperature"=w1924, "VSA_V2"=w1927, "VPI C3"=w1922, "Data Output C1"=w1932, "VPI C2"=w1921, "SN"=w1936, "R/W Status"=w1934, "Cap Header"=w1923, "HD/Cycles Completed"=w1928, "Data Output C2"=w1919, "VSA_V3"=w1925, "Current"=w1931, "VPI C1"=w1930, "Total Delta C3(pF)"=w1916) -> ("error out"=w1937:errorcluster)  [unwired: 2 in]
                  }
                  frame True {
                  }
                }
                n483 = case shown="True" "Debug" {
                  tunnel: w1865 -> [w1941 w1944]
                  tunnel: [w1941 w1942] -> w1864
                  frame False {
                  }
                  frame True {
                    n484 = Multiply(x=w1944, y="No of Rows\nFrom Spread Sheet") -> (x*y=w1942:i32)
                  }
                }
                n485 = Concatenate Strings(w1874, "\\" ("string"), w1868, "_Multi Socket Data.csv" ("string")) -> (w1873:string)
                n486 = local write "STATUS"(w1859) -> ()
              }
              frame #8 {
                n487 = case shown="True" "Plot Delta Cmin" {
                  tunnel: w1950 -> [w1964 w1979]
                  tunnel: [w1964 w1975] -> w1949
                  tunnel: w1948 -> [_ w1971]
                  tunnel: w1946 -> [_ w1969]
                  frame False {
                  }
                  frame True {
                    n488 = String To Path(string=w1971) -> (path=w1970:path)
                    n489 = call "Delay.vi"("milliseconds to wait"=u32 50, "error in (no error)"=w1979) -> ("error out"=w1978:errorcluster)  [unwired: 9 in]
                    n490 = call "36DUT Plot From Spread Sheet.vi"("Plot"="Plot", "No of Rows"=w1969, "error in (no error)"=w1978, "Bank"="Bank C1", "file path (dialog if empty)"=w1970) -> ("error out"=w1973:errorcluster, "Delta C_Min Plot"=→"Min Plot_1":dbl[][])  [unwired: 5 in]
                    n491 = call "36DUT Plot From Spread Sheet.vi"("Plot"="Plot", "No of Rows"=w1969, "error in (no error)"=w1973, "Bank"="Bank C2", "file path (dialog if empty)"=w1970) -> ("error out"=w1974:errorcluster, "Delta C_Min Plot"=→"Min Plot_2":dbl[][])  [unwired: 5 in]
                    n492 = call "36DUT Plot From Spread Sheet.vi"("Plot"="Plot", "No of Rows"=w1969, "error in (no error)"=w1974, "Bank"="Bank C3", "file path (dialog if empty)"=w1970) -> ("error out"=w1975:errorcluster, "Delta C_Min Plot"=→"Min Plot_3":dbl[][])  [unwired: 5 in]
                  }
                }
                n493 = Get Date/Time In Seconds() -> (seconds since 1Jan1904=w1957:timestamp)
                n494 = Get Date/Time String(seconds (now)=w1957, want seconds? (F)=TRUE) -> (date string=→"date string":string, time string=→"Previous Time":string)  [unwired: 1 in]
                n495 = Greater Or Equal?(x=w1954, y="Set HD/Cycle \nto Complete") -> (x >= y?=w1961:bool)
                n496 = Greater Or Equal?(x=w1953, y="TTF Completed") -> (x >= y?=w1952:bool)
                "No of HD/Cycle\nCompleted" <- w1954
              }
            }
            n497 = Increment(x=w600) -> (x+1=→"Loop \ncompleted":i32)
            n498 = call "Delay.vi"("milliseconds to wait"=u32 10, "error in (no error)"=w490) -> ("error out"=w491:errorcluster)  [unwired: 9 in]
            n499 = Compound Arithmetic op=OR(w669, w570, w596) -> (w609:bool)
          }
          "Total Time" <- w432
          n500 = Increment(x=w430) -> (x+1=→"Run Loops":i32)
          n501 = local write "No of HD/Cycle\nCompleted"(u64 0 ("No of HD/Cycle\nCompleted")) -> ()
          n502 = Unbundle By Name(w422) -> ("status"=w436:bool)
          n503 = Compound Arithmetic op=OR(w436, w428, w427) -> (w410:bool)
        }
        n504 = for {
          tunnel: w303 -> [w1991]
          tunnel: w282 -> [w1990]
          tunnel: w332 -> [w1988] mode=indexing
          tunnel: [w1983] -> w301
          tunnel: [w1987] -> w331
          n505 = call "E3631A_Voltage Controller updated.vi"("VISA resource name"=w1990, "I_VDD(A)"=0.5, "Channel Controller"=w1988, "Voltage 1"=0.0, "Voltage 2"=3.3, "error in (no error)"=w1991, "I_3.3V (A)"=0.5) -> ("VISA resource name out"=w1987:refnum<visa-resource-name>, "error out"=w1984:errorcluster)  [unwired: 7 in]
          n506 = call "Delay.vi"("milliseconds to wait"=u32 100, "error in (no error)"=w1984) -> ("error out"=w1983:errorcluster)  [unwired: 9 in]
        }
        n507 = VISA Write(VISA resource name=w322, write buffer="SOUR:FUNC VOLT;VOLT:MODE FIX;RANG 100;LEV 0.0;:SENS:FUNC \"CURR\";CURR:PROT 60E-3;RANG 100E-3;:OUTP ON", error in (no error)=w303) -> (VISA resource name out=w320:refnum<visa-resource-name>, error out=w302:errorcluster)  [unwired: 1 out]
        n508 = Merge Errors(w301, w302) -> (w321:errorcluster)
      }
      frame True {
      }
    }
    n509 = Wait Until Next ms Multiple(millisecond multiple=u32 100) -> ()  [unwired: 1 out]
    n510 = Unbundle By Name(w66) -> ("status"=w65:bool)
    n511 = Compound Arithmetic op=OR(w64, w65, w86) -> (w94:bool)
    "STATUS" <- "Idle...." ("STATUS")
  }
  "Ke2000 Out" <- w10
  n512 = local write "stop During HD/Cycles"(w16) -> ()
  n513 = local write "stop"(w16) -> ()
  n514 = case shown="True" w25 {
    tunnel: [w2008 w2011] -> w8
    tunnel: w4 -> [w2008 w2010]
    frame False {
    }
    frame True {
      n515 = local write "Online"(FALSE ("Online")) -> ()
      n516 = call "WSVCAP SHL Host TL Close.vi"("error in"=w2010) -> ("error out"=w2011:errorcluster)  [unwired: 14 in]
    }
  }
  "error out" <- w8
  n517 = VISA Write(VISA resource name=w20, write buffer="SOUR:FUNC VOLT;VOLT:MODE FIX;RANG 100;LEV 0.0;:SENS:FUNC \"CURR\";CURR:PROT 60E-3;RANG 100E-3;:OUTP OFF", error in (no error)=w4) -> (VISA resource name out=→"VISA resource name out":refnum<visa-resource-name>, error out=w7:errorcluster)  [unwired: 1 out]
  n518 = VISA Write(VISA resource name=w5, write buffer=":INST:NSEL 1; :VOLT 0.000000;:OUTP 1;", error in (no error)=w4) -> (VISA resource name out=→"PS1 Out":refnum<visa-resource-name>, error out=w3:errorcluster)  [unwired: 1 out]
  n519 = Merge Errors(w3, w8, w7) -> (→"error out 2":errorcluster)
